vi "eyecat MAX v01_Js.vi"() -> ()   [LabVIEW 2011]
doc: "This VI is an upgrade from the WIN 1_v4 that implements the ageing subrutine"
uses:
  Buttons/String output.ctl
  <vilib>/Utility/miscctls.llb/LVRowAndColumnTypeDef.ctl
  Buttons/Numeric control.ctl
  Buttons/String input.ctl
  Buttons/Numeric indicator.ctl
  Controls Win/Control 3.ctl
  <vilib>/Platform/TimedLoop/XDataNode/nitl_modes.ctl
  <vilib>/Platform/TimedLoop/XDataNode/timing_clust.ctl
  <vilib>/Platform/TimedLoop/XDataNode/wakeup.ctl
  <vilib>/Utility/file.llb/Write To Spreadsheet File (string).vi
  <vilib>/Utility/file.llb/Read From Spreadsheet File (string).vi
  <vilib>/Platform/TimedLoop/XDataNode/XDataNode.xnode
  <vilib>/regexp/Match Regular Expression.xnode
  <vilib>/Platform/TimedLoop/XDataNode/XDNodeRunTimeDep.lvlib
panel:
  out "Furnace temp 2":dbl
  out "output cluster":T2
  out "Full system?":bool
  out "Log interval (seconds)":T1
  in  "Flow rate Age":dbl
  in  "Inlet temp Age":dbl
  out "Stopped?":bool
  in  "Stop Cmd":T1
  out "Connected?":bool
  out "Error":dbl
  out "Iteration Duration":i64
  out "Finished Late? [i-1]":bool
  in  "stop TCP":bool
  in  "SO2 ppm":dbl
  out "Furnace temp 1":dbl
  out "stop 2":bool
  in  "Enum 1":i16=1
  in  "Acknowledge":bool
  out "Test number":u16
  out "Flag1":bool=TRUE
  out "EditPos Subc":T3
  out "Flag 2":bool=TRUE
  in  "Tab Control":T4(tab)
  out "Doors Unlocked":bool
  in  "Temperature Limit (°C)":T1=800.0 min=0.0 max=1200.0 step=1.0
  in  "Log Test Button":bool
  in  "File Name":T5
  in  "File Path":path=path "C:/DATA LOG"
  out "Fail":bool
  out "Pass":bool
  in  "Select Test Type":T6(radio)
  out "Standby":bool
  out "Doors Open":bool
  out "Extractor Fan On":bool
  out "Test In Progress":bool
  out "Cool Down":bool
  out "System Alarm":bool
  in  "Execute Leak Test Button":bool
  in  "Stop Test Button":bool
  in  "Start Test Button":bool
  in  "Advanced settings":bool
  in  "Inlet Temperature (°C)":T1=400.0 min=350.0 max=1000.0 step=1.0
  in  "Inlet LAMBDA Rich":T1=0.9 min=0.85 max=0.96 step=0.001
  in  "Inlet LAMBDA Lean":T1=1.2 min=1.02 max=3.0 step=0.001
  in  "Test Stop temperature (°C)":T1=300.0 min=100.0 max=1000.0 step=1.0
  in  "Test Start Temperature (°C)":T1=125.0 min=0.0 max=500.0 step=1.0
  in  "Furnace Ramp Rate (°C/min)":T1=15.0 min=1.0 max=50.0 step=0.1
  in  "NO:CO Ratio":T1=1.1 min=1.0 max=5.0 step=0.1
  in  "Inlet O2 (%)":T1=0.5 min=0.0 max=14.0 step=0.01
  in  "Inlet LAMBDA":T1=1.0 min=0.6 max=3.0 step=0.001
  out "Space Velocity (h-1)":T7
  out "Vol Flow @ STP (l/min)":T7
  in  "Test Flow Rate(g/s)":T1 min=0.0 max=100.0 step=0.01
  out "Sample Volume (litres)":T7
  in  "Number of Samples":T1=1.0 min=1.0 max=6.0 step=1.0
  in  "Sample Diameter (mm)":T1
  out "CO Theory (%)":T7 format="%#_3g"
  out "CO Theory (%)":T7 format="%#_3g"
  out "HC Theory (%)":T7
  in  "Sample Length (mm)":T1 min=0.0 step=0.5
  in  "NO ppm SW":dbl=500.0 caption="NO (ppm)" min=0.0 max=500.0 step=1.0
  in  "NO ppm Loff":T1 caption="NO ppm"
  in  "Delete sCycle":bool
  in  "Load sCycle":bool
  in  "Save sCycle":bool
  in  "Clear subcycle":bool
  in  "Clear Cycle Pattern":bool
  in  "Save Cycle":bool
  in  "Load Cycle":bool
  in  "Delete Cycle":bool
  out "Test Compiled":bool
  in  "Compile Test Button":bool
  in  "Sub-Cycle List":i32(listbox)=1
  in  "Cycle List":i32(listbox)=2
  out "Total Test Duration (hrs)":T8
  in  "Ageing Gas":enum32{"Radio Selection 1", "Radio Selection 2"}(radio)
  in  "Sub-Cycle Pattern":string[][](table) caption="Subcycle pattern"
  in  "Total Number of Cycles":T1=1.0 min=1.0 max=10000.0 step=1.0
  in  "Cycle Pattern":string[][](table)
  in  "Sub-Cycle Name":T5
  in  "Cycle Name":T5
  out "Heat Exchanger Temperatures (°C)":dynamicdata(graph)
  out "Flow Rate (g/s)":dynamicdata(graph)
  out "Sample Temperatures (°C)":dynamicdata(graph)
  out "System Temperatures (°C)":dynamicdata(graph)
  out "HC Concentration (ppm)":dynamicdata(graph)
  out "Lambda":dynamicdata(graph)
  out "M584L Upstream & Downstream":dynamicdata(graph)
  out "NO Concentration (ppm)":dynamicdata(graph)
  in  "Purge System":bool
  in  "Alarm ack":bool
  in  "Clear log":bool
  out "Table":string[][](table)
  out "Soft Alarm":bool
  out "Hard Alarm":bool
  # "Test Type"
  # "Test Commands"
  # "System Indicators"
  # "Leak Test"
  # "Catalyst Specification"
  # "Lightoff Settings"
  # "Furnace Lightoff Settings"
  # "Sweep Settings"
  # "CO/HC Lightoff Settings"
  # "0.96 < lambda < 0.85"
  # "1.02< lambda < 1.6"
  # "350 < Tinlet < 1000"
  # "NO Lightoff Settings"
  # "Flow Specification"
  # "Cycle Compiled"
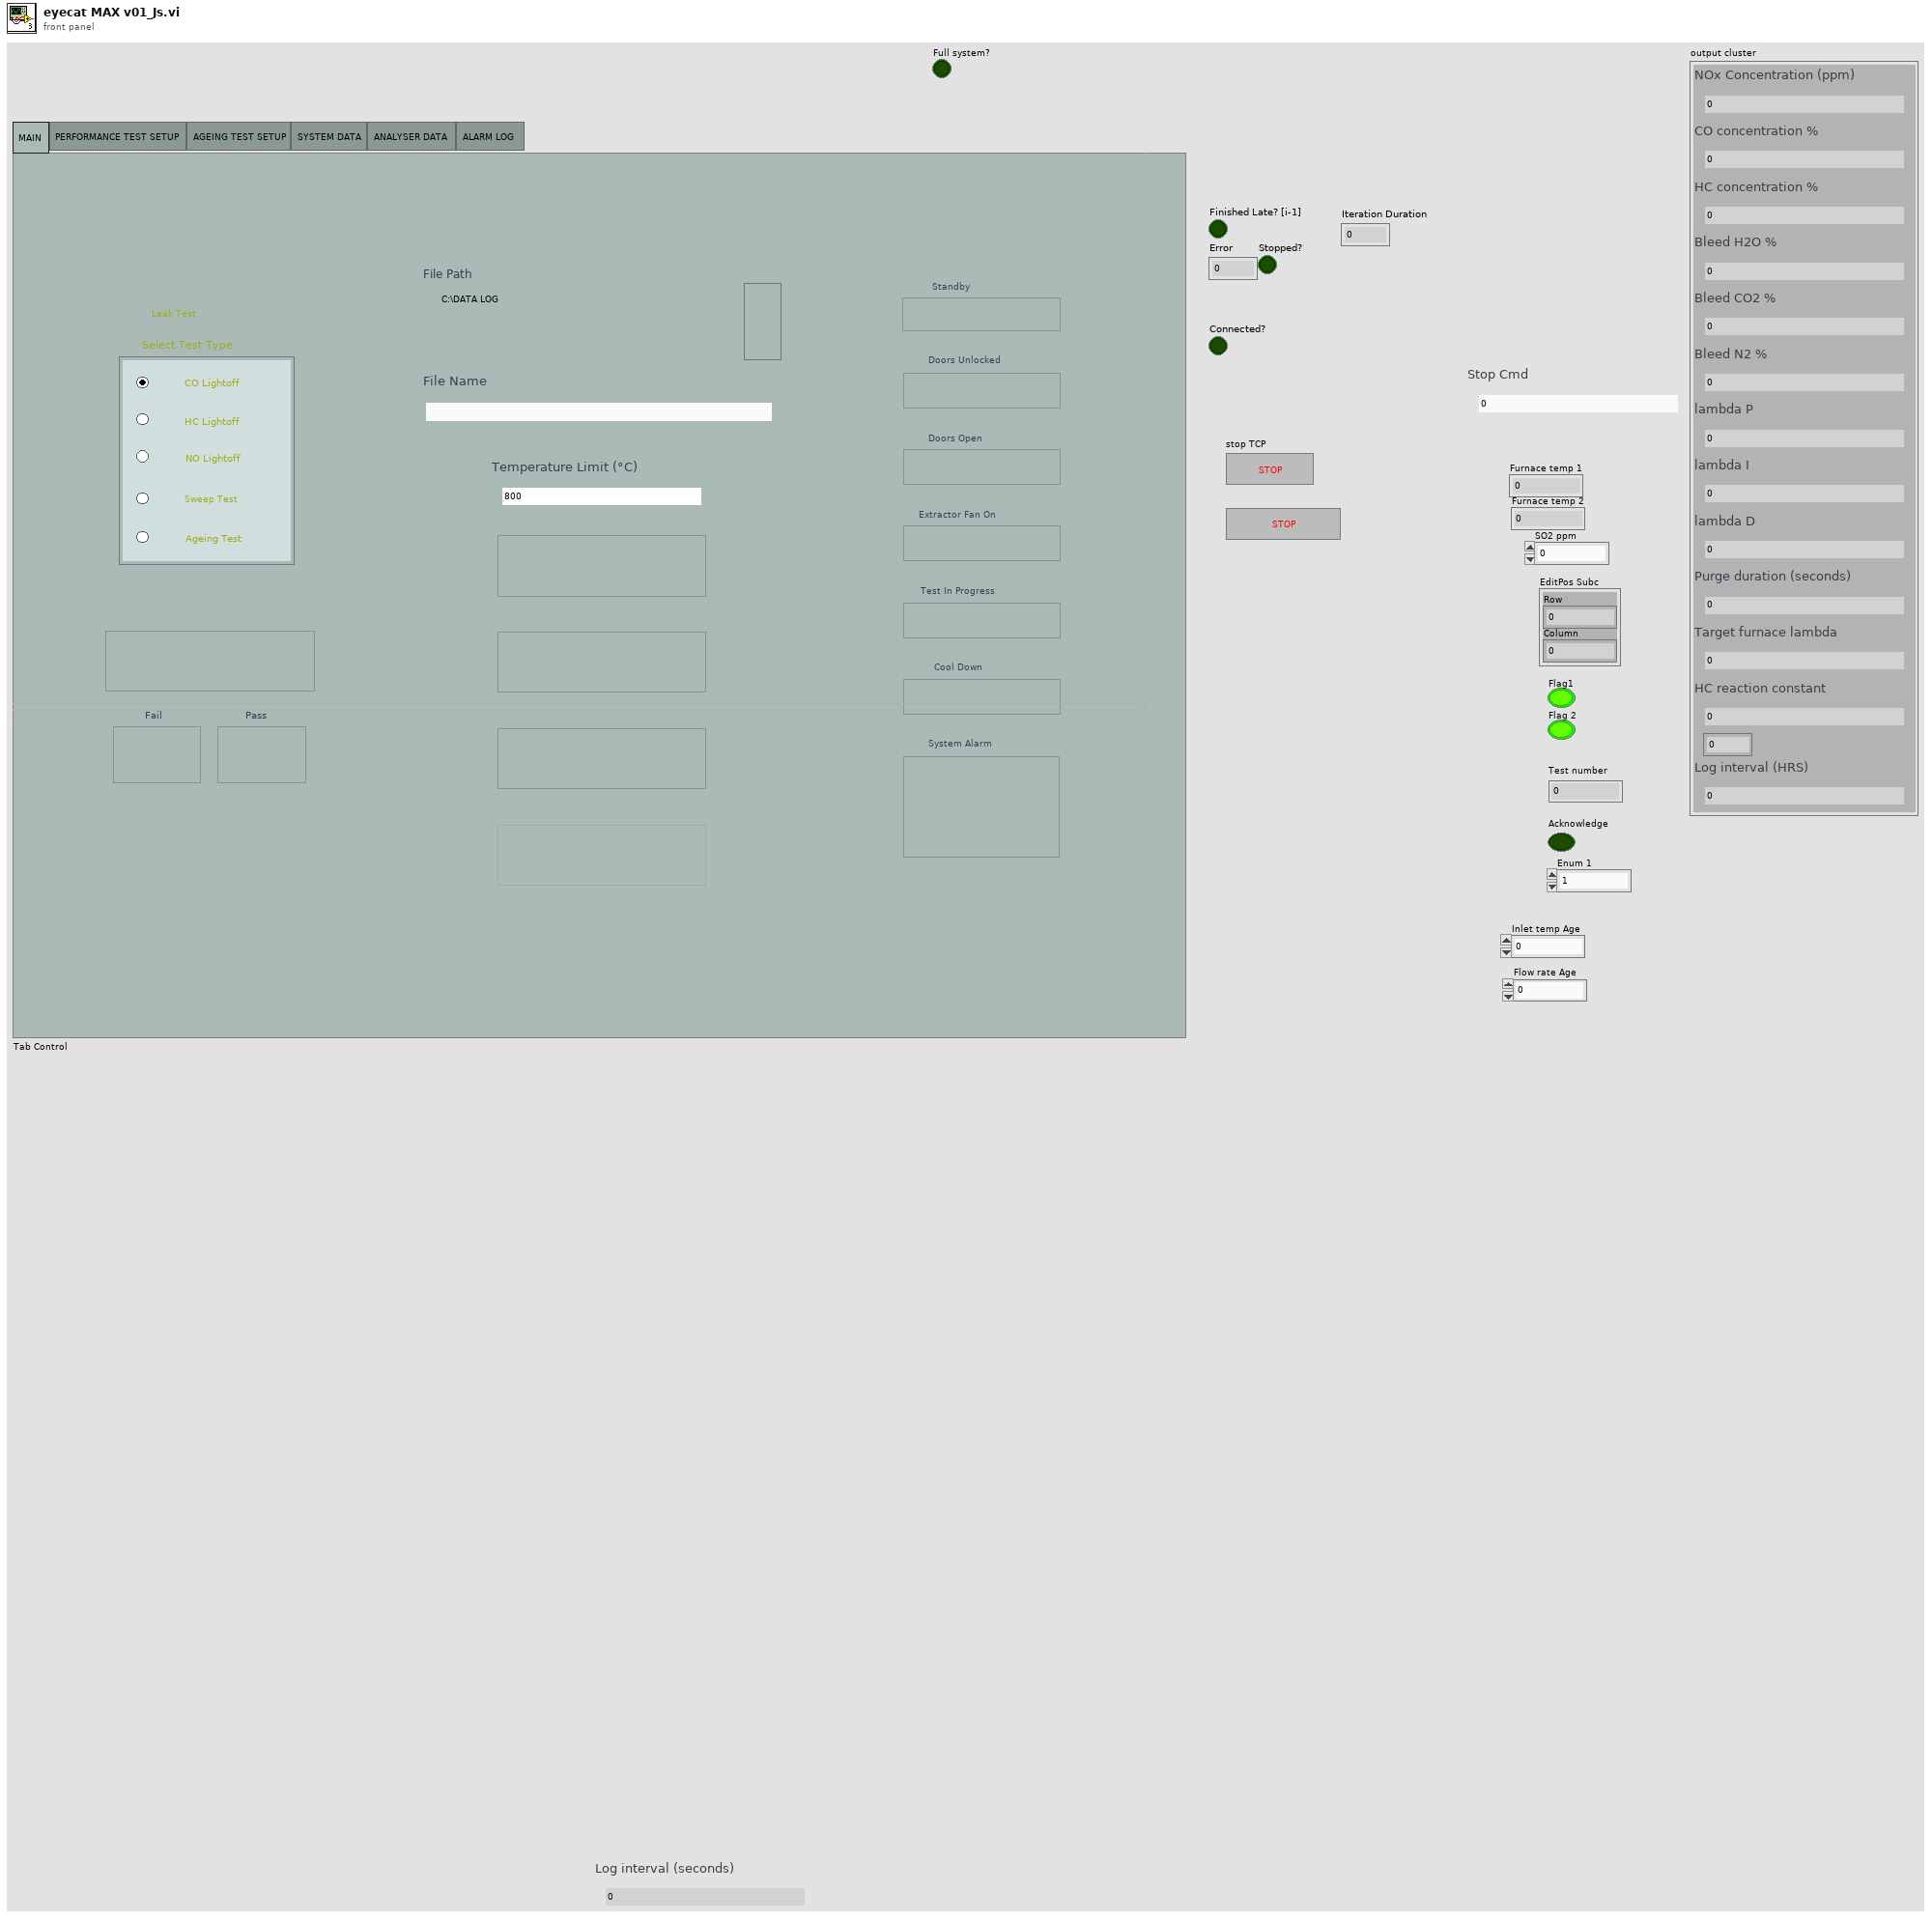
[diagram p1: front panel]
types:
  T1 = typedef "Numeric control.ctl" = dbl
  T2 = cluster{"NOx Concentration (ppm)":T1, "CO concentration %":T1, "HC concentration %":T1, "Bleed H2O %":T1, "Bleed CO2 %":T1, "Bleed N2 %":T1, "lambda P":T1, "lambda I":T1, "lambda D":T1, "Purge duration (seconds)":T1, "Target furnace lambda":T1, "HC reaction constant":T1, i16, "Log interval (HRS)":T1}
  T3 = typedef "LVRowAndColumnTypeDef.ctl" = cluster{"Row":i32, "Column":i32}
  T4 = enum32{"MAIN", "PERFORMANCE TEST SETUP", "AGEING TEST SETUP", "SYSTEM DATA", "ANALYSER DATA", "ALARM LOG"}
  T5 = typedef "String input.ctl" = string
  T6 = enum32{"CO Lightoff", "HC Lightoff", "NO Lightoff", "Sweep Test", "Ageing Test"}
  T7 = typedef "Numeric indicator.ctl" = dbl
  T8 = typedef "String output.ctl" = string
  T9 = typedef "XDNodeRunTimeDep.lvlib/nitl_modes.ctl" = enum32{"No Change", "Process missed periods, maintain original phase", "Discard missed periods, maintain original phase", "Process missed periods, ignore original phase", "Discard missed periods, ignore original phase"}
  T10 = typedef "Control 3.ctl" = enum16{"main", "start test", "save subc", "load subc", "delete subc", "clear table 1", "update list 1", "save cycle", "load cycle", "delete cycle", "clear table 2", "update list 2", "calc HC CO", "Total time calc", "update Cycle pattern ", "load cycle name", "convert to num", "load test array", "check scycle name", "check cycle name", "Multigas connect", "Multigas disconnect"}
  T11 = typedef "XDNodeRunTimeDep.lvlib/timing_clust.ctl" = cluster{"Expected End [f-1]":u64, "Actual End [f-1]":u64, "Finished Late? [f-1]":bool, "Expected End [i-1]":u64, "Actual End [i-1]":u64, "Finished Late? [i-1]":bool, "Expected Start [i]":u64, "Actual Start [i]":u64, "Expected Start [f]":u64, "Actual Start [f]":u64, "Source Name":string, "Structure Name":string, "Period":i64, "Deadline":i64, "Offset":i64, "Start":i64, "Priority":i32, "Timeout":i32, "Mode":T9, "Wakeup Reason":T12, "Error":errorcluster, "Source Type":string, "Secondary Source Type":string, "Global End Time":u64, "Global Start Time":u64, "Frame Duration":u64, "Iteration Duration":u64, "Assigned CPU":i32, "I/O Scan Engine Mode":u32}
  T12 = typedef "XDNodeRunTimeDep.lvlib/wakeup.ctl" = enum32{"Normal", "Aborted", "Asynchronous wakeup", "Timing source error", "Timed loop error", "Timeout"}
  T13 = enum8{"Enabled", "Disabled", "Disabled and Grayed Out"}
  T14 = cluster{"NOx Concentration (ppm)":T1, "CO concentration %":T1, "HC concentration %":T1, "Bleed H2O %":T1, "Bleed CO2 %":T1, "Bleed N2 %":T1, "lambda P":T1, "lambda I":T1, "lambda D":T1, "Purge duration (seconds)":T1, "Target furnace lambda":T1, "HC reaction constant":T1, "Full System?":i16, "Log interval (HRS)":T1}
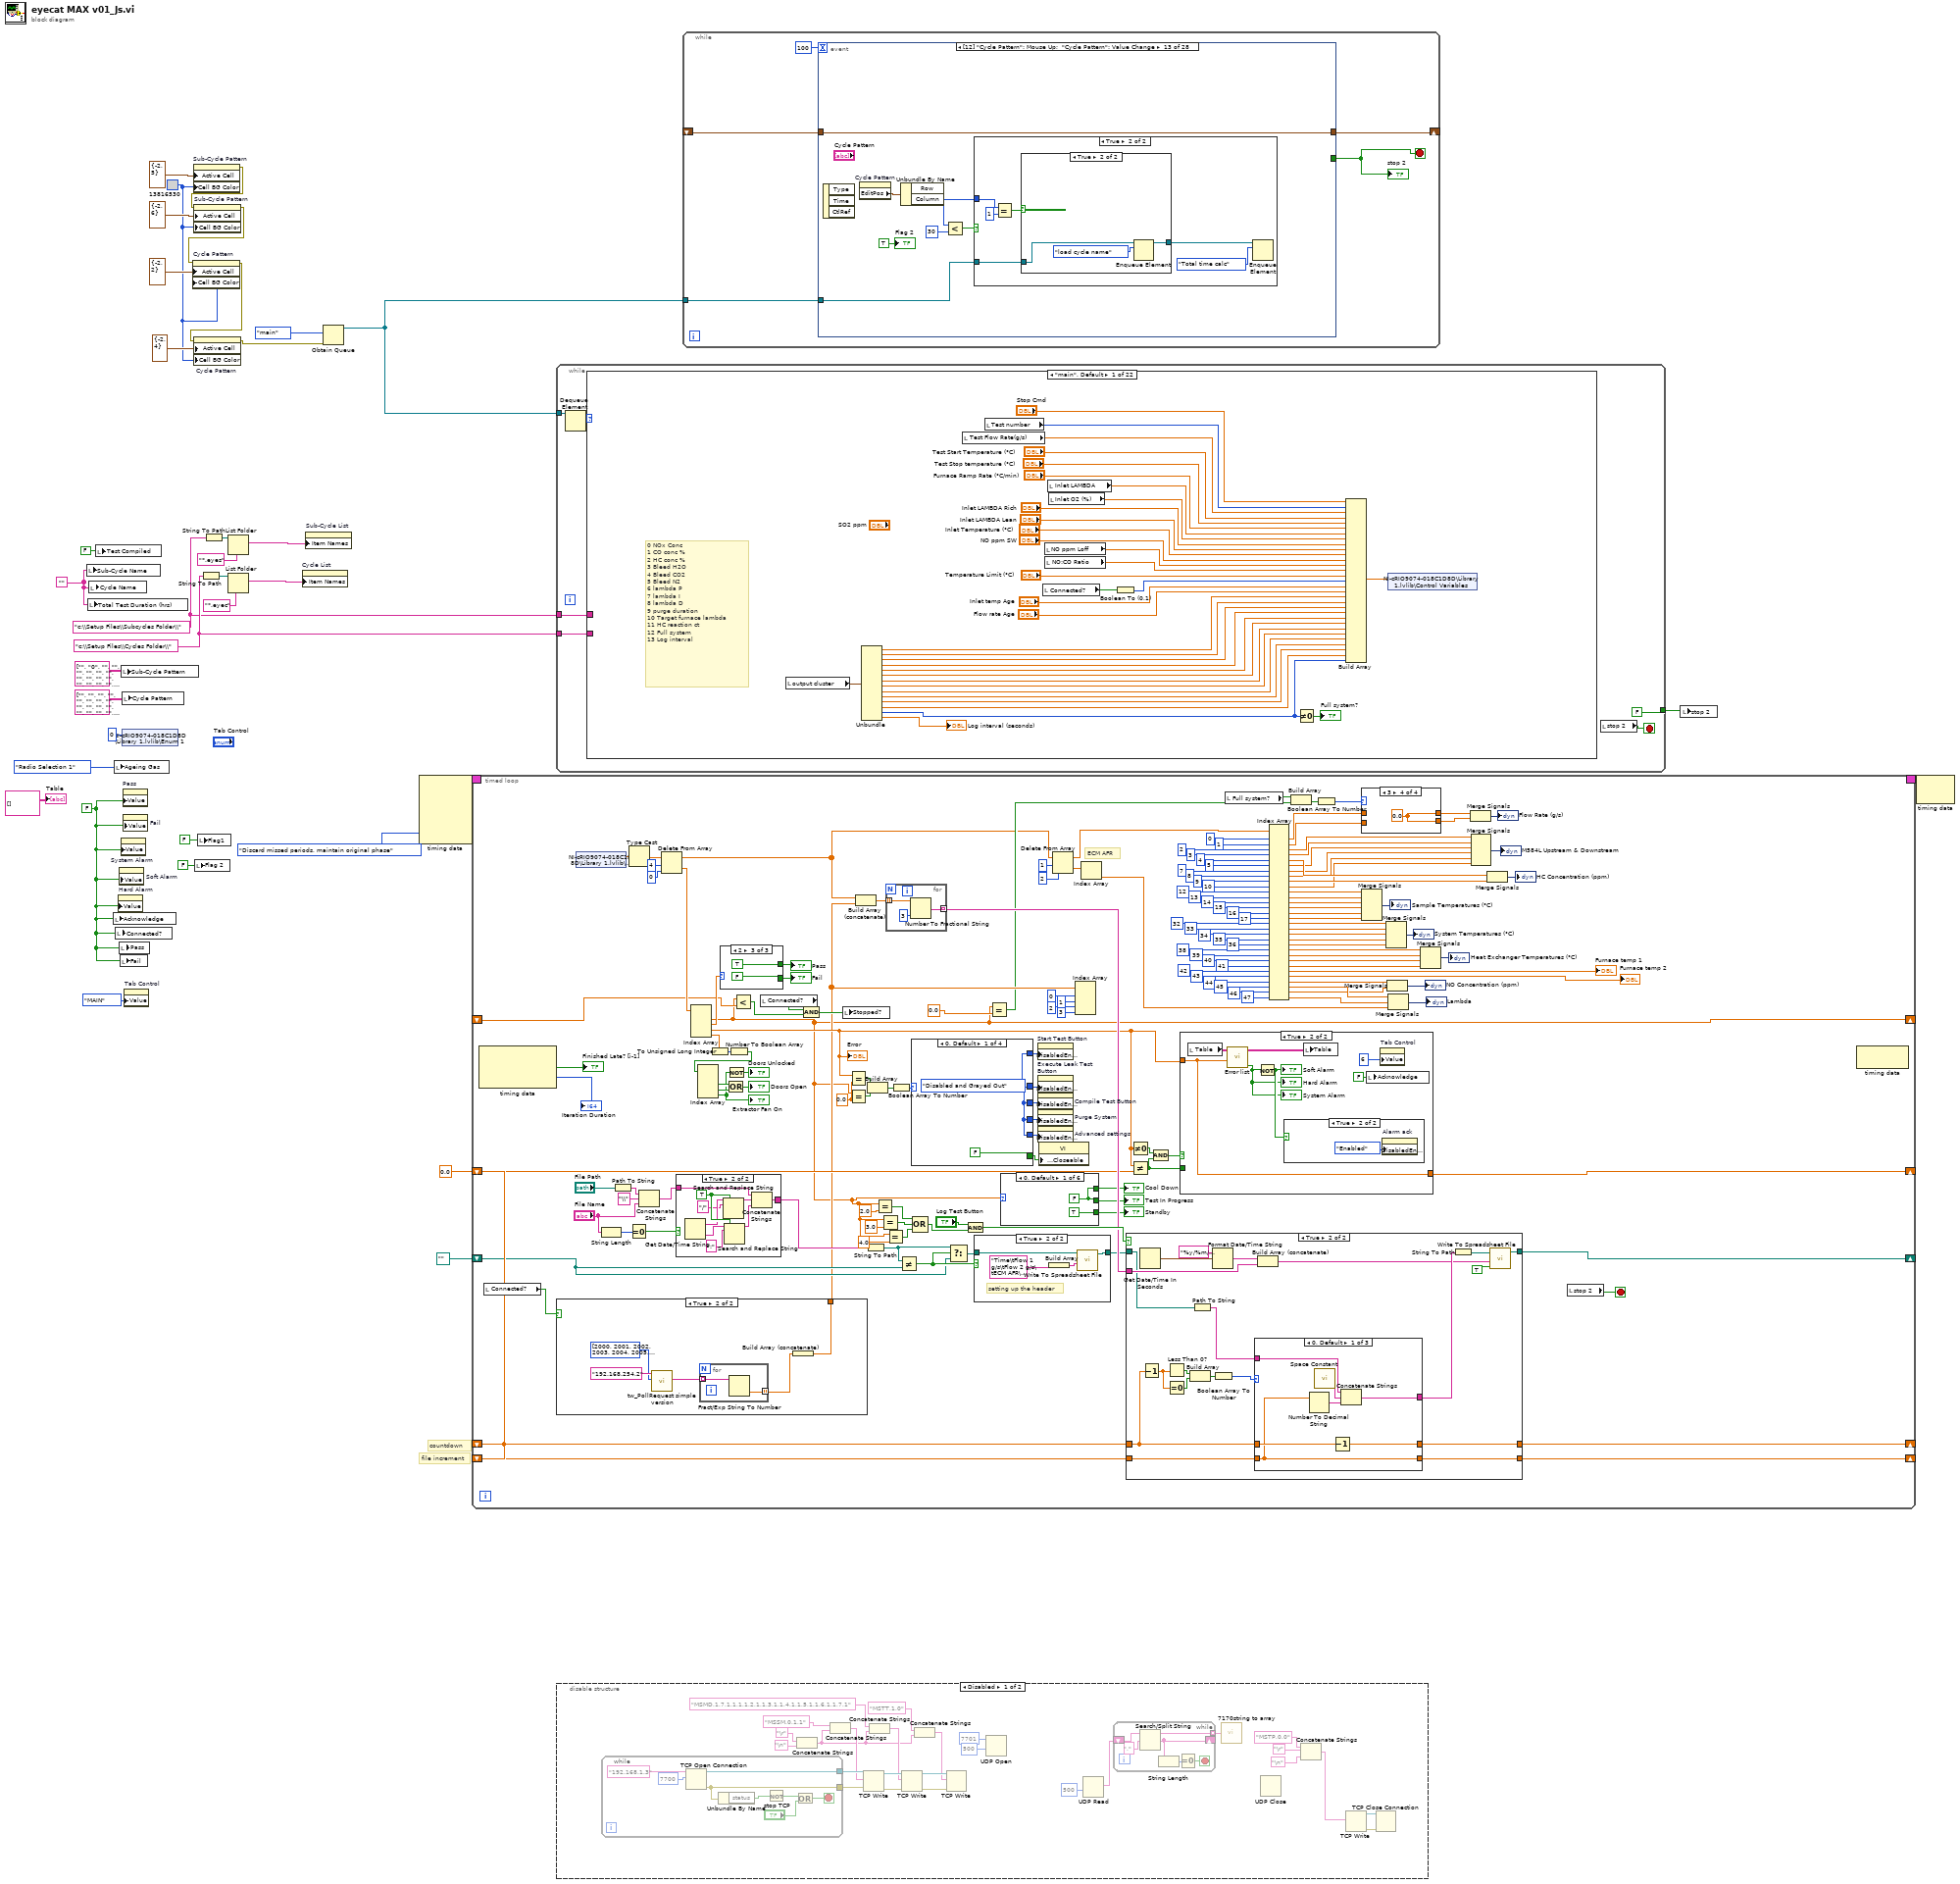
[diagram p0: block diagram]
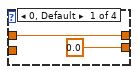
[diagram p3: hidden frame]
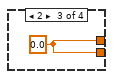
[diagram p5: hidden frame]
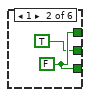
[diagram p7: hidden frame]
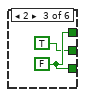
[diagram p8: hidden frame]
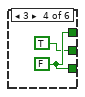
[diagram p9: hidden frame]
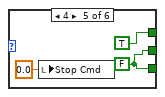
[diagram p10: hidden frame]
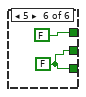
[diagram p11: hidden frame]
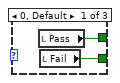
[diagram p12: hidden frame]
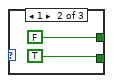
[diagram p13: hidden frame]
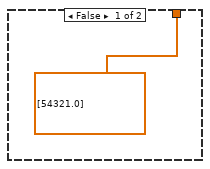
[diagram p14: hidden frame]
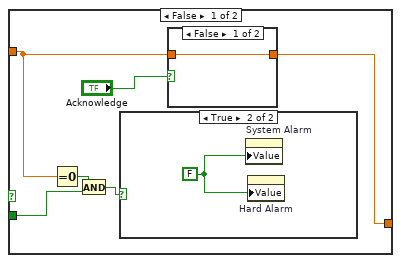
[diagram p15: hidden frame]
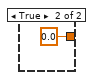
[diagram p16: hidden frame]
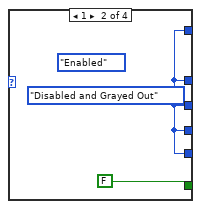
[diagram p19: hidden frame]
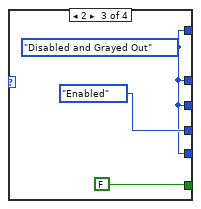
[diagram p20: hidden frame]
diagram:
  w2 = FALSE
  w1 = 0.0 ("y")
  w18 = ""
  w21 = "c:\\Setup Files\\Cycles Folder\\"
  w27 = u32 13816530
  w19 = "c:\\Setup Files\\Subcycles Folder\\"
  # "file increment"
  # "countdown"
  n1 = local write "Sub-Cycle Name"(w18) -> ()
  n2 = local write "Total Test Duration (hrs)"(w18) -> ()
  n3 = local write "Cycle Name"(w18) -> ()
  n4 = local write "Test Compiled"(FALSE ("Cycle Compiled")) -> ()
  n5 = local write "Acknowledge"(w2) -> ()
  n6 = local write "Ageing Gas"(enum32{"Radio Selection 1", "Radio Selection 2"}."Radio Selection 1" ("Ageing Gas")) -> ()
  n7 = local write "Connected?"(w2) -> ()
  n8 = property on="Hard Alarm" class="Bool (strict)"("Value"=w2) -> ()  [unwired: 2 in, 2 out]
  n9 = property on="Soft Alarm" class="Bool (strict)"("Value"=w2) -> ()  [unwired: 2 in, 2 out]
  n10 = local write "Pass"(w2) -> ()
  n11 = local write "Fail"(w2) -> ()
  n12 = local write "Sub-Cycle Pattern"(string[][] [["", "0", "", "", "", "", "", "", "", "", "", "", ""], ["", "", "", "", "", "", "", "", "", "", "", "", ""], ["", "", "", "", "", "", "", "", "", "", "", "", ""], ["", "", "", "", "", "", "", "", "", "", "", "", ""], ["", "", "", "", "", "", "", "", "", "", "", "", ""], ["", "", "", "", "", "", "", "", "", "", "", "", ""], ["", "", "", "", "", "", "", "", "", "", "", "", ""], ["", "", "", "", "", "", "", "", "", "", "", "", ""], ["", "", "", "", "", "", "", "", "", "", "", "", ""], ["", "", "", "", "", "", "", "", "", "", "", "", ""], ["", "", "", "", "", "", "", "", "", "", "", "", ""], ["", "", "", "", "", "", "", "", "", "", "", "", ""], ["", "", "", "", "", "", "", "", "", "", "", "", ""], ["", "", "", "", "", "", "", "", "", "", "", "", ""], ["", "", "", "", "", "", "", "", "", "", "", "", ""], ["", "", "", "", "", "", "", "", "", "", "", "", ""], ["", "", "", "", "", "", "", "", "", "", "", "", ""], ["", "", "", "", "", "", "", "", "", "", "", "", ""], ["", "", "", "", "", "", "", "", "", "", "", "", ""], ["", "", "", "", "", "", "", "", "", "", "", "", ""], ["", "", "", "", "", "", "", "", "", "", "", "", ""], ["", "", "", "", "", "", "", "", "", "", "", "", ""], ["", "", "", "", "", "", "", "", "", "", "", "", ""], ["", "", "", "", "", "", "", "", "", "", "", "", ""], ["", "", "", "", "", "", "", "", "", "", "", "", ""], ["", "", "", "", "", "", "", "", "", "", "", "", ""], ["", "", "", "", "", "", "", "", "", "", "", "", ""], ["", "", "", "", "", "", "", "", "", "", "", "", ""], ["", "", "", "", "", "", "", "", "", "", "", "", ""], ["", "", "", "", "", "", "", "", "", "", "", "", ""], ["", "", "", "", "", "", "", "", "", "", "", "", ""]]) -> ()
  n13 = property on="System Alarm" class="Bool (strict)"("Value"=w2) -> ()  [unwired: 2 in, 2 out]
  n14 = local write "Cycle Pattern"(string[][] [["", "", "", "", ""], ["", "", "", "", ""], ["", "", "", "", ""], ["", "", "", "", ""], ["", "", "", "", ""], ["", "", "", "", ""], ["", "", "", "", ""], ["", "", "", "", ""], ["", "", "", "", ""], ["", "", "", "", ""], ["", "", "", "", ""], ["", "", "", "", ""], ["", "", "", "", ""], ["", "", "", "", ""], ["", "", "", "", ""], ["", "", "", "", ""], ["", "", "", "", ""], ["", "", "", "", ""], ["", "", "", "", ""], ["", "", "", "", ""], ["", "", "", "", ""], ["", "", "", "", ""], ["", "", "", "", ""], ["", "", "", "", ""], ["", "", "", "", ""], ["", "", "", "", ""], ["", "", "", "", ""], ["", "", "", "", ""], ["", "", "", "", ""], ["", "", "", "", ""], ["", "", "", "", ""]]) -> ()
  n15 = shared-variable "NI-cRIO9074-018C1D8D\\Library 1.lvlib\\Enum 1"(u16 0 ("Enum 1")) -> ()  [unwired: 1 in, 1 out]
  n16 = property on="Pass" class="Bool (strict)"("Value"=w2) -> ()  [unwired: 2 in, 2 out]
  n17 = property on="Fail" class="Bool (strict)"("Value"=w2) -> ()  [unwired: 2 in, 2 out]
  n18 = property on="Tab Control" class="TabCtl (strict)"("Value"=T4."MAIN" ("Tab Control")) -> ()  [unwired: 2 in, 2 out]
  n19 = property on="Sub-Cycle Pattern" class="Tbl (strict)"("Active Cell"=T3 {"Row"=-2, "Column"=5} ("Active Cell:Active Cell"), "Cell BG Color"=w27) -> (error out=w32:errorcluster)  [unwired: 2 in, 1 out]
  n20 = property on="Sub-Cycle Pattern" class="Tbl (strict)"(error in=w32, "Active Cell"=T3 {"Row"=-2, "Column"=6} ("Active Cell:Active Cell"), "Cell BG Color"=w27) -> (error out=w31:errorcluster)  [unwired: 1 in, 1 out]
  n21 = property on="Cycle Pattern" class="Tbl (strict)"(error in=w31, "Active Cell"=T3 {"Row"=-2, "Column"=2} ("Active Cell:Active Cell"), "Cell BG Color"=w27) -> (error out=w29:errorcluster)  [unwired: 1 in, 1 out]
  n22 = property on="Cycle Pattern" class="Tbl (strict)"(error in=w29, "Active Cell"=T3 {"Row"=-2, "Column"=4} ("Active Cell:Active Cell"), "Cell BG Color"=w27) -> (error out=w26:errorcluster)  [unwired: 1 in, 1 out]
  n23 = local write "Flag 2"(FALSE) -> ()
  n24 = local write "Flag1"(FALSE) -> ()
  n25 = String To Path(string=w21) -> (path=w22:path)
  n26 = String To Path(string=w19) -> (path=w24:path)
  n27 = List Folder(path=w22, pattern="*.eyec") -> (filenames=w23:string[])  [unwired: 2 in, 3 out]
  n28 = List Folder(path=w24, pattern="*.eyes") -> (filenames=w25:string[])  [unwired: 2 in, 3 out]
  n29 = property on="Cycle List" class="LstBox (strict)"("Item Names"=w23) -> ()  [unwired: 2 in, 2 out]
  n30 = property on="Sub-Cycle List" class="LstBox (strict)"("Item Names"=w25) -> ()  [unwired: 2 in, 2 out]
  n31 = Obtain Queue(element data type=Control_3."main" ("Enum"), error in (no error)=w26) -> (queue out=w35:refnum<queue>)  [unwired: 3 in, 2 out]
  n32 = node-c288(nitl_modes."Discard missed periods, maintain original phase" ("Mode")) -> (w7:T11)  [unwired: 4 in]
  n33 = timed-loop {
    timing: w7 -> [_]
    timing-out: [_] -> w6
    shift-right: [w168] -> _
    shift-left: path "" -> [w170]
    shift-right: [w119] -> _
    shift-left: w1 -> [w169]
    shift-right: [w38] -> _
    shift-left: _ -> [w133]
    shift-right: [w108] -> _
    shift-left: w1 -> [w112]
    shift-right: [w109] -> _
    shift-left: w1 -> [w111]
    stop <- w167 stop-if-true
    w150 = 0.0 ("y")
    # "ECM AFR"
    n34 = node-c288() -> (→"Finished Late? [i-1]":bool, →"Iteration Duration":i64)  [unwired: 1 in, 1 out]
    n35 = local read "Connected?"() -> (w156:bool)
    n36 = case shown="True" w156 {
      tunnel: [dbl[] [54321.0] ("Output") w235] -> w107
      frame False {
      }
      frame True {
        n37 = call <userlib>:"tw_PollRequest simple version.vi"("EVID list"=i32[] [2000, 2001, 2002, 2003, 2004, 2005, 2006, 2007, 2008, 2009, 2010, 2011, 2012, 2013, 2014], "IP_ADD [127.0.0.1]"="192.168.254.2") -> ("values out"=w239:string[])  [unwired: 7 in, 2 out]
        n38 = for {
          tunnel: [w241] -> w236 mode=indexing
          tunnel: w239 -> [w240] mode=indexing
          n39 = Fract/Exp String To Number(string=w240) -> (number=w241:dbl)  [unwired: 3 in, 1 out]
        }
        n40 = Build Array (concatenate)(w236) -> (w235:dbl[])
      }
    }
    n41 = shared-variable "NI-cRIO9074-018C1D8D\\Library 1.lvlib\\DATA"() -> (w166:dbl[])  [unwired: 1 in, 1 out]
    n42 = String Length(string="File Name") -> (length=w124:i32)
    n43 = Path To String(path="File Path") -> (string=w126:string)
    n44 = Equal To 0?(x=w124) -> (x = 0?=w122:bool)
    n45 = Type Cast(type=w166, x=w166) -> (*(type *) &x=w179:dbl[])
    n46 = Concatenate Strings(w126, "\\" ("string"), "File Name") -> (w121:string)
    n47 = Delete From Array(array=w179, length=4, index=0) -> (deleted portion=w176:dbl[], array with subset deleted=w48:dbl[])
    n48 = case shown="True" w122 {
      tunnel: [w205 w213] -> w110
      tunnel: w121 -> [w205 w214]
      frame False {
      }
      frame True {
        w211 = TRUE ("replace all? (F)")
        n49 = Get Date/Time String() -> (date string=w209:string, time string=w210:string)  [unwired: 3 in]
        n50 = Search and Replace String(replace all?=w211, input string=w209, search string="/") -> (result string=w212:string)  [unwired: 5 in, 3 out]
        n51 = Search and Replace String(replace all?=w211, input string=w210, search string=":") -> (result string=w206:string)  [unwired: 5 in, 3 out]
        n52 = Concatenate Strings(w214, w212, w206) -> (w213:string)
      }
    }
    n53 = Index Array(array=w176) -> (element #1=w38:dbl, element #2=w139:dbl, element #3=w140:dbl, element #4=w132:dbl)  [unwired: 4 in]
    "Error" <- w140
    n54 = To Unsigned Long Integer(number=w132) -> (unsigned 32bit integer=w131:u32)
    n55 = case shown="2" w139 {
      tunnel: [w228 TRUE FALSE] -> w138
      tunnel: [w229 FALSE TRUE] -> w137
      frame 0, Default {
        n56 = local read "Pass"() -> (w229:bool)
        n57 = local read "Fail"() -> (w228:bool)
      }
      frame 1 {
      }
      frame 2 {
      }
    }
    "Pass" <- w137
    "Fail" <- w138
    n58 = Number To Boolean Array(number=w131) -> (Boolean array=w155:bool[])
    n59 = Index Array(array=w155) -> (element #2=w153:bool, element #3=w152:bool, element #4=w128:bool)  [unwired: 4 in, 1 out]
    "Extractor Fan On" <- w128
    n60 = Or(x=w153, y=w152) -> (x .or. y?=→"Doors Open":bool)
    n61 = Not(x=w128) -> (.not. x?=→"Doors Unlocked":bool)
    n62 = Less?(x=w38, y=w133) -> (x < y?=w130:bool)
    n63 = local read "Connected?"() -> (w129:bool)
    n64 = And(x=w129, y=w130) -> (x .and. y?=w118:bool)
    n65 = local write "Stopped?"(w118) -> ()
    n66 = Equal?(x=w140, y=w150) -> (x = y?=w148:bool)
    n67 = Equal?(x=w38, y=w150) -> (x = y?=w147:bool)
    n68 = Build Array (concatenate)(w48, w107) -> (w172:dbl[])
    n69 = String To Path(string=w110) -> (path=w120:path)
    n70 = Build Array(w148, w147) -> (w146:bool[])
    n71 = Equal?(x=w38, y=2.0) -> (x = y?=w50:bool)
    n72 = Equal?(x=w38, y=3.0) -> (x = y?=w41:bool)
    n73 = Equal?(x=w38, y=4.0) -> (x = y?=w39:bool)
    n74 = for {
      tunnel: w172 -> [w274] mode=indexing
      tunnel: [w273] -> w183 mode=indexing
      n75 = Number To Fractional String(number=w274, precision (6)=i16 3) -> (F-format string=w273:string)  [unwired: 2 in]
    }
    n76 = Boolean Array To Number(Boolean array=w146) -> (number=w145:u32)
    n77 = Not Equal?(x=w120, y=w170) -> (x != y?=w181:bool)
    n78 = case shown="0, Default" w145 {
      tunnel: [w260 w262 w264 w267] -> w149
      tunnel: [w260 w262 w264 w267] -> w144
      tunnel: [w260 w262 w264 w267] -> w143
      tunnel: [w260 w262 T13."Enabled" ("Disabled") w267] -> w142
      tunnel: [w260 w262 w264 w267] -> w141
      tunnel: [FALSE FALSE FALSE TRUE] -> w117
      frame 0, Default {
        w260 = T13."Disabled and Grayed Out" ("Disabled")
      }
      frame 1 {
        (unwired) T13."Enabled" ("Disabled")
        w262 = T13."Disabled and Grayed Out" ("Disabled")
      }
      frame 2 {
        w264 = T13."Disabled and Grayed Out" ("Disabled")
      }
      frame 3 {
        w267 = T13."Enabled" ("Disabled")
        (unwired) T13."Disabled and Grayed Out" ("Disabled")
      }
    }
    n79 = Compound Arithmetic op=OR(w50, w41, w39) -> (w49:bool)
    n80 = Select(t=w120, s=w181, f=w170) -> (s? t:f=w182:path)
    n81 = And(x="Log Test Button", y=w49) -> (x .and. y?=w198:bool)
    n82 = case shown="True" w181 {
      tunnel: w182 -> [w268 w272]
      tunnel: [w268 w271] -> w180
      frame False {
      }
      frame True {
        # "setting up the header"
        n83 = Build Array("Time\tFlow 1 g/s\tFlow 2 g/s\tECM AFR\tCO2 U %\tCO U %\tHC U ppm\tO2 U %\tNO U ppm\tCO2 D %\tCO D %\tHC D ppm\tO2 D %\tNO D ppm\tTC1X\tTC2A\tTCY\tTC4B\tTC5\tTC6\tTC7\tTC8\tTC9\tTC10\tTC11\tTC12\tTC13\tTC14\tTC15\tTC16\tTC17\tTC18\tTC19\tTC20\tTC Vent 1\tTC Vent 2\tTC Fan B1\tTC Fan B2\tTC Cab\tTC Ex A\tTC Ex B\tTC Ex C\tTC Ex D\tTC Furn 1\tTC Furn 2\tNOX 1 ppm\tNLambda 1\tNOX 2 ppm\tNLambda 2\tEGO 1\tEGO 2\tEGO 3\tEGO 4\tCO2 U %\tCO U %\tHC U ppm\tO2 U %\tNO U ppm\tCO2 D %\tCO D %\tHC D ppm\tO2 D %\tNO D ppm\r\n" ("Heading string 2")) -> (w270:string[])
        n84 = call-poly <vilib>:"Write To Spreadsheet File.vi"("1D data"=w270, "file path (dialog if empty)"=w272) -> ("new file path (Not A Path if cancelled)"=w271:path)  [unwired: 6 in]
      }
    }
    n85 = Equal?(x=w38, y=0.0) -> (x = y?=w104:bool)
    n86 = case shown="0, Default" w38 {
      tunnel: [w215 w218 w220 w222 TRUE FALSE] -> w136
      tunnel: [w215 TRUE TRUE TRUE w224 w226] -> w135
      tunnel: [TRUE w218 w220 w222 w224 w226] -> w134
      frame 0, Default {
        w215 = FALSE
      }
      frame 1 {
        w218 = FALSE
      }
      frame 2 {
        w220 = FALSE
      }
      frame 3 {
        w222 = FALSE
      }
      frame 4 {
        w224 = FALSE
        n87 = local write "Stop Cmd"(T1 0.0 ("Stop Cmd")) -> ()
      }
      frame 5 {
        w226 = FALSE
      }
    }
    "Cool Down" <- w136
    "Test In Progress" <- w135
    "Standby" <- w134
    n88 = property on="Start Test Button" class="Bool"("DisabledEnum"=w149) -> ()  [unwired: 2 in, 2 out]
    n89 = property on="Execute Leak Test Button" class="Bool"("DisabledEnum"=w144) -> ()  [unwired: 2 in, 2 out]
    n90 = property on="Compile Test Button" class="Bool"("DisabledEnum"=w143) -> ()  [unwired: 2 in, 2 out]
    n91 = property on="Purge System" class="Bool"("DisabledEnum"=w142) -> ()  [unwired: 2 in, 2 out]
    n92 = property on="Advanced settings" class="Bool"("DisabledEnum"=w141) -> ()  [unwired: 2 in, 2 out]
    n93 = property class="VI"("Front Panel.Closeable"=w117) -> ()  [unwired: 2 in, 2 out]
    n94 = Delete From Array(array=w48, length=1, index=2) -> (deleted portion=w45:dbl[], array with subset deleted=w43:dbl[])
    n95 = Index Array(array=w107, index #1=0 ("index"), index #2=1 ("index"), index #3=2 ("index"), index #4=3 ("index")) -> ()  [unwired: 4 out]
    n96 = Index Array(array=w45) -> (element=w44:dbl)  [unwired: 1 in]
    n97 = case shown="True" w198 {
      tunnel: w180 -> [w278 w286]
      tunnel: [w278 w298] -> w168
      tunnel: w183 -> [_ w294]
      tunnel: w112 -> [_ w287]
      tunnel: w111 -> [w277 w282]
      tunnel: [w277 w284] -> w109
      tunnel: [w276 w283] -> w108
      frame False {
        n98 = local read "Log interval (seconds)"() -> (w276:T1)
      }
      frame True {
        n99 = Get Date/Time In Seconds() -> (seconds since 1Jan1904=w295:timestamp)
        n100 = Decrement(x=w287) -> (x-1=w288:T1)
        n101 = Less Than 0?(x=w288) -> (x < 0?=w289:bool)
        n102 = Equal To 0?(x=w288) -> (x = 0?=w290:bool)
        n103 = Build Array(w289, w290) -> (w291:bool[])
        n104 = Path To String(path=w286) -> (string=w281:string)
        n105 = Format Date/Time String(time format string (%c)="%y/%m/%d %H:%M:%S", seconds (now)=w295) -> (date/time string=w296:string)  [unwired: 1 in]
        n106 = Boolean Array To Number(Boolean array=w291) -> (number=w292:u32)
        n107 = case shown="0, Default" w292 {
          tunnel: w287 -> [w305 w306 _]
          tunnel: [w304 w306 w309] -> w283
          tunnel: w281 -> [w303 w308 w312]
          tunnel: [w300 w308 w310] -> w285
          tunnel: [w299 w307 w311] -> w284
          tunnel: w282 -> [w299 w307 w315]
          frame 0, Default {
            n108 = Number To Decimal String(number=w299) -> (decimal integer string=w301:string)  [unwired: 1 in]
            n109 = call <vilib>:"Space Constant.vi"() -> ("String"=w302:string)
            n110 = Decrement(x=w305) -> (x-1=w304:T1)
            n111 = Concatenate Strings(w303, w302, w301) -> (w300:string)
          }
          frame 1 {
          }
          frame 2 {
            n112 = local read "Log interval (seconds)"() -> (w309:T1)
            n113 = Increment(x=w315) -> (x+1=w311:dbl)
            n114 = Number To Decimal String(number=w311) -> (decimal integer string=w313:string)  [unwired: 1 in]
            n115 = call <vilib>:"Space Constant.vi"() -> ("String"=w314:string)
            n116 = Concatenate Strings(w312, w314, w313) -> (w310:string)
          }
        }
        n117 = Build Array (concatenate)(w296, w294) -> (w280:string[])
        n118 = String To Path(string=w285) -> (path=w279:path)
        n119 = call-poly <vilib>:"Write To Spreadsheet File.vi"("append to file? (new file:F)"=TRUE, "1D data"=w280, "file path (dialog if empty)"=w279) -> ("new file path (Not A Path if cancelled)"=w298:path)  [unwired: 5 in]
      }
    }
    n120 = Not Equal To 0?(x=w140) -> (x != 0?=w174:bool)
    n121 = Not Equal?(x=w140, y=w169) -> (x != y?=w173:bool)
    n122 = And(x=w174, y=w173) -> (x .and. y?=w175:bool)
    n123 = case shown="True" w175 {
      tunnel: w140 -> [w243 w254]
      tunnel: w173 -> [w246 _]
      tunnel: [w242 w254] -> w119
      frame False {
        n124 = Equal To 0?(x=w243) -> (x = 0?=w247:bool)
        n125 = And(x=w247, y=w246) -> (x .and. y?=w245:bool)
        n126 = case shown="True" w245 {
          frame False {
          }
          frame True {
            w250 = FALSE ("Ack hard alarm!")
            n127 = property on="System Alarm" class="Bool (strict)"("Value"=w250) -> ()  [unwired: 2 in, 2 out]
            n128 = property on="Hard Alarm" class="Bool (strict)"("Value"=w250) -> ()  [unwired: 2 in, 2 out]
          }
        }
        n129 = case shown="False" "Acknowledge" {
          tunnel: [w248 0.0 ("Numeric")] -> w242
          tunnel: w243 -> [w248 _]
          frame False {
          }
          frame True {
          }
        }
      }
      frame True {
        n130 = local read "Table"() -> (w257:string[][])
        n131 = call "Error list.vi"("Error code"=w254, "Error array in"=w257) -> ("Hard alarm?"=w251:bool, "Error array out"=w256:string[][])  [unwired: 8 in]
        "Hard Alarm" <- w251
        "System Alarm" <- w251
        n132 = Not(x=w251) -> (.not. x?=w252:bool)
        "Soft Alarm" <- w252
        n133 = case shown="True" w252 {
          frame False {
          }
          frame True {
            n134 = property on="Alarm ack" class="Bool"("DisabledEnum"=T13."Enabled" ("Disabled")) -> ()  [unwired: 2 in, 2 out]
          }
        }
        n135 = local write "Table"(w256) -> ()
        n136 = local write "Acknowledge"(FALSE ("Acknowledge")) -> ()
        n137 = property on="Tab Control" class="TabCtl (strict)"("Value"=6) -> ()  [unwired: 2 in, 2 out]
      }
    }
    n138 = local read "Full system?"() -> (w105:bool)
    n139 = Index Array(array=w43, index #1=0 ("index"), index #2=1 ("index"), index #3=2 ("index"), index #4=3 ("index"), index #5=4 ("index"), index #6=5 ("index"), index #7=7 ("index"), index #8=8 ("index"), index #9=9 ("index"), index #10=10 ("index"), index #11=12 ("index"), index #12=13 ("index"), index #13=14 ("index"), index #14=15 ("index"), index #15=16 ("index"), index #16=17 ("index"), index #17=32 ("index"), index #18=33 ("index"), index #19=34 ("index"), index #20=35 ("index"), index #21=36 ("index"), index #22=38 ("index"), index #23=39 ("index"), index #24=40 ("index"), index #25=41 ("index"), index #26=42 ("index"), index #27=43 ("index"), index #28=44 ("index"), index #29=45 ("index"), index #30=46 ("index"), index #31=47 ("index")) -> (element #1=w102:dbl, element #2=w101:dbl, element #3=w98:dbl, element #4=w96:dbl, element #5=w97:dbl, element #6=w95:dbl, element #7=w94:dbl, element #8=w93:dbl, element #9=w92:dbl, element #10=w91:dbl, element #11=w86:dbl, element #12=w85:dbl, element #13=w84:dbl, element #14=w83:dbl, element #15=w82:dbl, element #16=w81:dbl, element #17=w75:dbl, element #18=w74:dbl, element #19=w73:dbl, element #20=w72:dbl, element #21=w71:dbl, element #22=w66:dbl, element #23=w65:dbl, element #24=w64:dbl, element #25=w63:dbl, element #26=→"Furnace temp 1":dbl, element #27=→"Furnace temp 2":dbl, element #28=w56:dbl, element #29=w55:dbl, element #30=w52:dbl, element #31=w51:dbl)
    n140 = Build Array(w105, w104) -> (w106:bool[])
    n141 = Boolean Array To Number(Boolean array=w106) -> (number=w103:u32)
    n142 = case shown="3" w103 {
      tunnel: w102 -> [w200 w202 _ _]
      tunnel: w101 -> [_ w201 _ _]
      tunnel: [w200 w202 w203 w204] -> w100
      tunnel: [0.0 ("y") w201 w203 w204] -> w99
      frame 0, Default {
      }
      frame 1 {
      }
      frame 2 {
        w203 = 0.0 ("y")
      }
      frame 3 {
        w204 = 0.0 ("y")
      }
    }
    n143 = Merge Signals(w86, w85, w84, w83, w82, w81) -> (→"Sample Temperatures (°C)":dynamicdata)
    n144 = Merge Signals(w75, w74, w73, w72, w71) -> (→"System Temperatures (°C)":dynamicdata)
    n145 = Merge Signals(w56, w52) -> (→"NO Concentration (ppm)":dynamicdata)
    n146 = Merge Signals(w55, w51, w44) -> (→"Lambda":dynamicdata)
    n147 = Merge Signals(w66, w65, w64, w63) -> (→"Heat Exchanger Temperatures (°C)":dynamicdata)
    n148 = Merge Signals(w100, w99) -> (→"Flow Rate (g/s)":dynamicdata)
    n149 = Merge Signals(w98, w96, w95, w94, w93, w91) -> (→"M584L Upstream & Downstream":dynamicdata)
    n150 = Merge Signals(w97, w92) -> (→"HC Concentration (ppm)":dynamicdata)
    n151 = local read "stop 2"() -> (w167:bool)
    n152 = node-c288() -> ()  [unwired: 1 in, 1 out]
  }
  n153 = while {
    tunnel: w35 -> [w324]
    tunnel: w19 -> [w322]
    tunnel: w21 -> [w321]
    tunnel: [FALSE ("stop 2")] -> w9
    stop <- w325 stop-if-true
    n154 = Dequeue Element(queue=w324) -> (element=w323:T10)  [unwired: 2 in, 3 out]
    n155 = case shown="\"main\", Default" w323 {
      tunnel: w322 -> [_ _ _ w370 w381 w417 w451 _ _ _ _ _ _ _ w814 _ _ _ _ _ _ _]
      tunnel: w321 -> [_ _ _ _ _ _ _ _ w464 w479 w534 w579 _ _ _ _ _ _ _ _ _ _]
      frame "main", Default {
        # "0 NOx Conc\n1 CO conc %\n2 HC conc %\n3 Bleed H2O \n4 Bleed CO2\n5 Bleed N2 \n6 lambda P\n7 lambda I\n8 lambda D\n9 purge duration\n10 Target furnace lambda\n11 HC reaction ct\n12 Full system\n13 Log interval"
        n156 = local read "output cluster"() -> (w344:T2)
        n157 = Unbundle(w344) -> ("NOx Concentration (ppm)"=w330:T1, "CO concentration %"=w329:T1, "HC concentration %"=w328:T1, "Bleed H2O %"=w327:T1, "Bleed CO2 %"=w326:T1, "Bleed N2 %"=w341:T1, "lambda P"=w340:T1, "lambda I"=w339:T1, "lambda D"=w342:T1, "Purge duration (seconds)"=w343:T1, "Target furnace lambda"=w335:T1, "HC reaction constant"=w334:T1, w336:i16, "Log interval (HRS)"=→"Log interval (seconds)":T1)
        n158 = local read "Test Flow Rate(g/s)"() -> (w356:T1)
        n159 = local read "Test number"() -> (w361:u16)
        n160 = local read "Connected?"() -> (w350:bool)
        n161 = local read "NO ppm Loff"() -> (w346:T1)
        n162 = local read "NO:CO Ratio"() -> (w345:T1)
        n163 = local read "Inlet LAMBDA"() -> (w348:T1)
        n164 = local read "Inlet O2 (%)"() -> (w347:T1)
        n165 = Boolean To (0,1)(Boolean=w350) -> (0, 1=w333:i16)
        n166 = Not Equal To 0?(x=w336) -> (x != 0?=→"Full system?":bool)
        n167 = Build Array("Stop Cmd", w361, w356, "Test Start Temperature (°C)", "Test Stop temperature (°C)", "Furnace Ramp Rate (°C/min)", w348, w347, "Inlet LAMBDA Rich", "Inlet LAMBDA Lean", "Inlet Temperature (°C)", "NO ppm SW", w346, w345, "Temperature Limit (°C)", w333, "Inlet temp Age", "Flow rate Age", w330, w329, w328, w327, w326, w341, w340, w339, w342, w343, w335, w334, w336) -> (w352:T1[])
        n168 = shared-variable "NI-cRIO9074-018C1D8D\\Library 1.lvlib\\Control Variables"(w352) -> ()  [unwired: 1 in, 1 out]
      }
      frame "start test" {
        w362 = FALSE
        n169 = property on="Pass" class="Bool (strict)"("Value"=w362) -> ()  [unwired: 2 in, 2 out]
        n170 = property on="Fail" class="Bool (strict)"("Value"=w362) -> ()  [unwired: 2 in, 2 out]
        n171 = local write "Pass"(w362) -> ()
        n172 = local write "Fail"(w362) -> ()
        n173 = shared-variable "NI-cRIO9074-018C1D8D\\Library 1.lvlib\\Enum 1"("Enum 1") -> ()  [unwired: 1 in, 1 out]
      }
      frame "clear table 1" {
        n174 = property on="Sub-Cycle Name" class="Str"("Value"="" ("Subcycle name")) -> ()  [unwired: 2 in, 2 out]
        n175 = local write "Flag1"(FALSE) -> ()
        n176 = local write "Sub-Cycle Pattern"(string[][] [["", "0", "", "", "", "", "", "", "", "", "", "", ""], ["", "", "", "", "", "", "", "", "", "", "", "", ""], ["", "", "", "", "", "", "", "", "", "", "", "", ""], ["", "", "", "", "", "", "", "", "", "", "", "", ""], ["", "", "", "", "", "", "", "", "", "", "", "", ""], ["", "", "", "", "", "", "", "", "", "", "", "", ""], ["", "", "", "", "", "", "", "", "", "", "", "", ""], ["", "", "", "", "", "", "", "", "", "", "", "", ""], ["", "", "", "", "", "", "", "", "", "", "", "", ""], ["", "", "", "", "", "", "", "", "", "", "", "", ""], ["", "", "", "", "", "", "", "", "", "", "", "", ""], ["", "", "", "", "", "", "", "", "", "", "", "", ""], ["", "", "", "", "", "", "", "", "", "", "", "", ""], ["", "", "", "", "", "", "", "", "", "", "", "", ""], ["", "", "", "", "", "", "", "", "", "", "", "", ""], ["", "", "", "", "", "", "", "", "", "", "", "", ""], ["", "", "", "", "", "", "", "", "", "", "", "", ""], ["", "", "", "", "", "", "", "", "", "", "", "", ""], ["", "", "", "", "", "", "", "", "", "", "", "", ""], ["", "", "", "", "", "", "", "", "", "", "", "", ""], ["", "", "", "", "", "", "", "", "", "", "", "", ""], ["", "", "", "", "", "", "", "", "", "", "", "", ""], ["", "", "", "", "", "", "", "", "", "", "", "", ""], ["", "", "", "", "", "", "", "", "", "", "", "", ""], ["", "", "", "", "", "", "", "", "", "", "", "", ""], ["", "", "", "", "", "", "", "", "", "", "", "", ""], ["", "", "", "", "", "", "", "", "", "", "", "", ""], ["", "", "", "", "", "", "", "", "", "", "", "", ""], ["", "", "", "", "", "", "", "", "", "", "", "", ""], ["", "", "", "", "", "", "", "", "", "", "", "", ""], ["", "", "", "", "", "", "", "", "", "", "", "", ""]]) -> ()
      }
      frame "update list 1" {
        n177 = String To Path(string=w370) -> (path=w369:path)
        n178 = List Folder(path=w369, pattern="*.eyes") -> (filenames=w368:string[])  [unwired: 2 in, 3 out]
        n179 = property on="Sub-Cycle List" class="LstBox (strict)"("Item Names"=w368) -> ()  [unwired: 2 in, 2 out]
      }
      frame "save subc" {
        w374 = ".eyes" ("string")
        n180 = local read "Sub-Cycle Name"() -> (w373:T5)
        n181 = String To Path(string=w381) -> (path=w386:path)
        n182 = Equal?(x=w373, y="") -> (x = y?=w378:bool)
        n183 = List Folder(path=w386, pattern="*.eyes" ("string")) -> (filenames=w385:string[])  [unwired: 2 in, 3 out]
        n184 = Concatenate Strings(w373, w374) -> (w372:string)
        n185 = Concatenate Strings(w381, w373, w374) -> (w387:string)
        n186 = Search 1D Array(1D array=w385, element=w372) -> (index of element=w384:i32)  [unwired: 1 in]
        n187 = case shown="True" w378 {
          tunnel: [TRUE FALSE] -> w377
          frame False {
          }
          frame True {
            n188 = One Button Dialog(message="Insert file name!") -> ()  [unwired: 1 in, 1 out]
          }
        }
        n189 = String To Path(string=w387) -> (path=w380:path)
        n190 = Equal?(x=w384, y=-1) -> (x = y?=w382:bool)
        n191 = case shown="False" w382 {
          selector: w382 -> [_ w393]
          tunnel: [w391 w393] -> w376
          frame False {
            n192 = Two Button Dialog(message="A file with this name already exists!\nDo you want to overwrite?") -> (T button?=w391:bool)  [unwired: 2 in]
          }
          frame True {
          }
        }
        n193 = And(x=w376, y=w377) -> (x .and. y?=w375:bool)
        n194 = case shown="True" w375 {
          tunnel: w380 -> [_ w398]
          frame False {
          }
          frame True {
            n195 = local read "Sub-Cycle Pattern"() -> (w397:string[][])
            n196 = call "Table check.vi"("Input table"=w397) -> ("Incomplete?"=w395:bool, "Length"=w396:i32)  [unwired: 9 in]
            n197 = case shown="False" w395 {
              tunnel: w397 -> [w406 _]
              tunnel: w398 -> [w405 _]
              tunnel: w396 -> [w404 _]
              tunnel: string[] [] -> [w403 _]
              frame False {
                n198 = for {
                  N: w404 -> [_]
                  tunnel: w406 -> [w413]
                  shift-right: [w410] -> w402
                  shift-left: w403 -> [w411]
                  i -> [w412]
                  n199 = Index Array(array=w413, index (row)=w412) -> (element=w409:string[])  [unwired: 1 in]
                  n200 = Delete From Array(array=w409, index=0) -> (array with subset deleted=w408:string[])  [unwired: 1 in, 1 out]
                  n201 = Build Array (concatenate)(w411, w408) -> (w410:string[])
                }
                n202 = Build Array (concatenate)("SubCycle Data File for EYECAT - do not modify", w402) -> (w400:string[])
                n203 = call-poly <vilib>:"Write To Spreadsheet File.vi"("1D data"=w400, "file path (dialog if empty)"=w405) -> ()  [unwired: 6 in, 1 out]
              }
              frame True {
                n204 = One Button Dialog(message="The table is incomplete!\nplease review and save again!") -> ()  [unwired: 1 in, 1 out]
              }
            }
            n205 = local write "Flag1"(FALSE) -> ()
          }
        }
      }
      frame "load subc" {
        n206 = local read "Flag1"() -> (w418:bool)
        n207 = case shown="True" w418 {
          tunnel: [w445 w447] -> w416
          tunnel: w417 -> [w445 w447]
          tunnel: [TRUE w446] -> w415
          frame False {
          }
          frame True {
            n208 = Two Button Dialog(message="The table has been modified.\nDo you want to continue?") -> (T button?=w446:bool)  [unwired: 2 in]
          }
        }
        n209 = case shown="True" w415 {
          tunnel: w416 -> [_ w422]
          frame False {
          }
          frame True {
            n210 = property on="Sub-Cycle List" class="LstBox (strict)"() -> ("Item Names"=w434:string[])  [unwired: 2 in, 2 out]
            n211 = Index Array(array=w434, index="Sub-Cycle List") -> (element=w421:string)
            n212 = Concatenate Strings(w422, w421) -> (w432:string)
            n213 = Search/Split String(string=w421, search string/char (-)=".") -> (substring before match=w419:string)  [unwired: 1 in, 2 out]
            n214 = local write "Sub-Cycle Name"(w419) -> ()
            n215 = String To Path(string=w432) -> (path=w431:path)
            n216 = call-poly <vilib>:"Read From Spreadsheet File.vi"("file path (dialog if empty)"=w431) -> ("first row"=w427:string[])  [unwired: 6 in, 4 out]
            n217 = Delete From Array(array=w427, length=1, index=0) -> (array with subset deleted=w424:string[])  [unwired: 1 out]
            n218 = Array Size(array=w424) -> (size(s)=w430:i32)
            n219 = Divide(x=w430, y=12) -> (x/y=w423:dbl)
            n220 = for {
              N: w423 -> [_]
              shift-right: [w440] -> _
              shift-left: w424 -> [w443]
              tunnel: [w439] -> w428 mode=indexing
              i -> [w438]
              n221 = Increment(x=w438) -> (x+1=w437:i32)
              n222 = Delete From Array(array=w443, length=12, index=0) -> (deleted portion=w435:string[], array with subset deleted=w440:string[])
              n223 = Number To Decimal String(number=w437) -> (decimal integer string=w436:string)  [unwired: 1 in]
              n224 = Build Array (concatenate)(w436, w435) -> (w439:string[])
            }
            n225 = local write "Sub-Cycle Pattern"(w428) -> ()
          }
        }
      }
      frame "delete subc" {
        n226 = Two Button Dialog(message="This operation will permanently delete this file!\nDo you want to continue?") -> (T button?=w450:bool)  [unwired: 2 in]
        n227 = case shown="True" w450 {
          tunnel: w451 -> [_ w456]
          frame False {
          }
          frame True {
            n228 = local read "Sub-Cycle List"() -> (w453:i32)
            n229 = property on="Sub-Cycle List" class="LstBox (strict)"() -> ("Item Names"=w454:string[])  [unwired: 2 in, 2 out]
            n230 = Index Array(array=w454, index=w453) -> (element=w458:string)
            n231 = Concatenate Strings(w456, w458) -> (w457:string)
            n232 = local write "Flag1"(FALSE) -> ()
            n233 = String To Path(string=w457) -> (path=w455:path)
            n234 = Delete(path (use dialog)=w455) -> ()  [unwired: 4 in, 3 out]
          }
        }
      }
      frame "clear table 2" {
        n235 = property on="Cycle Name" class="Str"("Value"="" ("Subcycle name")) -> ()  [unwired: 2 in, 2 out]
        n236 = local write "Flag 2"(FALSE) -> ()
        n237 = local write "Cycle Pattern"(string[][] [["", "", "", "", ""], ["", "", "", "", ""], ["", "", "", "", ""], ["", "", "", "", ""], ["", "", "", "", ""], ["", "", "", "", ""], ["", "", "", "", ""], ["", "", "", "", ""], ["", "", "", "", ""], ["", "", "", "", ""], ["", "", "", "", ""], ["", "", "", "", ""], ["", "", "", "", ""], ["", "", "", "", ""], ["", "", "", "", ""], ["", "", "", "", ""], ["", "", "", "", ""], ["", "", "", "", ""], ["", "", "", "", ""], ["", "", "", "", ""], ["", "", "", "", ""], ["", "", "", "", ""], ["", "", "", "", ""], ["", "", "", "", ""], ["", "", "", "", ""], ["", "", "", "", ""], ["", "", "", "", ""], ["", "", "", "", ""], ["", "", "", "", ""], ["", "", "", "", ""], ["", "", "", "", ""]]) -> ()
      }
      frame "update list 2" {
        n238 = String To Path(string=w464) -> (path=w465:path)
        n239 = List Folder(path=w465, pattern="*.eyec") -> (filenames=w463:string[])  [unwired: 2 in, 3 out]
        n240 = property on="Cycle List" class="LstBox (strict)"("Item Names"=w463) -> ()  [unwired: 2 in, 2 out]
      }
      frame "save cycle" {
        w466 = ".eyec" ("string")
        n241 = local read "Cycle Name"() -> (w467:T5)
        n242 = String To Path(string=w479) -> (path=w480:path)
        n243 = List Folder(path=w480, pattern="*.eyec" ("string")) -> (filenames=w478:string[])  [unwired: 2 in, 3 out]
        n244 = Equal?(x=w467, y="") -> (x = y?=w473:bool)
        n245 = Concatenate Strings(w467, w466) -> (w469:string)
        n246 = Search 1D Array(1D array=w478, element=w469) -> (index of element=w477:i32)  [unwired: 1 in]
        n247 = Concatenate Strings(w479, w467, w466) -> (w482:string)
        n248 = case shown="True" w473 {
          tunnel: [TRUE FALSE] -> w471
          frame False {
          }
          frame True {
            n249 = One Button Dialog(message="Insert file name!") -> ()  [unwired: 1 in, 1 out]
          }
        }
        n250 = String To Path(string=w482) -> (path=w481:path)
        n251 = Equal?(x=w477, y=-1) -> (x = y?=w475:bool)
        n252 = case shown="False" w475 {
          selector: w475 -> [_ w531]
          tunnel: [w529 w531] -> w472
          frame False {
            n253 = Two Button Dialog(message="A file with this name already exists!\nDo you want to overwrite?") -> (T button?=w529:bool)  [unwired: 2 in]
          }
          frame True {
          }
        }
        n254 = And(x=w472, y=w471) -> (x .and. y?=w470:bool)
        n255 = case shown="True" w470 {
          tunnel: w481 -> [_ w489]
          frame False {
          }
          frame True {
            n256 = local read "Cycle Pattern"() -> (w488:string[][])
            n257 = call "Table check.vi"("Input table"=w488) -> ("Incomplete?"=w486:bool, "Length"=w487:i32)  [unwired: 9 in]
            n258 = case shown="False" w486 {
              tunnel: w489 -> [w498 _]
              tunnel: w488 -> [w497 _]
              tunnel: w487 -> [w490 _]
              frame False {
                n259 = Number To Decimal String(number=w490) -> (decimal integer string=w493:string)  [unwired: 1 in]
                n260 = for {
                  N: w490 -> [_]
                  tunnel: w497 -> [w527]
                  shift-right: [w515] -> w494
                  shift-left: string[] [] -> [w525]
                  i -> [w526]
                  w506 = 12 ("length")
                  n261 = Index Array(array=w527, index (row)=w526) -> (element=w521:string[])  [unwired: 1 in]
                  n262 = Index Array(array=w521, index=3) -> (element=w511:string)
                  n263 = Index Array(array=w521, index=1) -> (element=w510:string)
                  n264 = Concatenate Strings("C:\\Setup Files\\Subcycles Folder\\", w510) -> (w522:string)
                  n265 = String To Path(string=w522) -> (path=w523:path)
                  n266 = call-poly <vilib>:"Read From Spreadsheet File.vi"("file path (dialog if empty)"=w523) -> ("first row"=w514:string[])  [unwired: 6 in, 4 out]
                  n267 = Delete From Array(array=w514, length=1, index=0) -> (array with subset deleted=w508:string[])  [unwired: 1 out]
                  n268 = String Length(string=w508) -> (length=w517:i32[])
                  n269 = Array Size(array=w517) -> (size(s)=w509:i32)
                  n270 = Divide(x=w509, y=w506) -> (x/y=w507:dbl)
                  n271 = Decrement(x=w507) -> (x-1=w499:dbl)
                  n272 = Multiply(x=w506, y=w499) -> (x*y=w505:dbl)
                  n273 = Number To Decimal String(number=w499) -> (decimal integer string=w516:string)  [unwired: 1 in]
                  n274 = Delete From Array(array=w508, length=12, index=w505) -> (deleted portion=w502:string[], array with subset deleted=w503:string[])
                  n275 = Index Array(array=w502, index=0) -> (element=w500:string)
                  n276 = Build Array (concatenate)(w510, w511, w516, w500, w503) -> (w520:string[])
                  n277 = Build Array (concatenate)(w525, w520) -> (w515:string[])
                }
                n278 = local write "Flag 2"(FALSE) -> ()
                n279 = Build Array (concatenate)("Cycle Data File for EYECAT - do not modify", w493, w494) -> (w495:string[])
                n280 = call-poly <vilib>:"Write To Spreadsheet File.vi"("1D data"=w495, "file path (dialog if empty)"=w498) -> ()  [unwired: 6 in, 1 out]
              }
              frame True {
                n281 = One Button Dialog(message="The table is incomplete!\nplease review and save again!") -> ()  [unwired: 1 in, 1 out]
              }
            }
          }
        }
      }
      frame "load cycle" {
        n282 = local read "Flag 2"() -> (w535:bool)
        n283 = case shown="True" w535 {
          tunnel: [w574 w576] -> w532
          tunnel: w534 -> [w574 w576]
          tunnel: [TRUE ("T button?") w575] -> w533
          frame False {
          }
          frame True {
            n284 = Two Button Dialog(message="The table has been modified.\nDo you want to continue?") -> (T button?=w575:bool)  [unwired: 2 in]
          }
        }
        n285 = case shown="True" w533 {
          tunnel: w532 -> [_ w538]
          frame False {
          }
          frame True {
            n286 = property on="Cycle List" class="LstBox (strict)"() -> ("Item Names"=w554:string[])  [unwired: 2 in, 2 out]
            n287 = Index Array(array=w554, index="Cycle List") -> (element=w540:string)
            n288 = Concatenate Strings(w538, w540) -> (w553:string)
            n289 = Search/Split String(string=w540, search string/char (-)=".") -> (substring before match=w539:string)  [unwired: 1 in, 2 out]
            n290 = String To Path(string=w553) -> (path=w552:path)
            n291 = local write "Cycle Name"(w539) -> ()
            n292 = call-poly <vilib>:"Read From Spreadsheet File.vi"("file path (dialog if empty)"=w552) -> ("first row"=w536:string[])  [unwired: 6 in, 4 out]
            n293 = Delete From Array(array=w536, length=2, index=0) -> (array with subset deleted=w537:string[])  [unwired: 1 out]
            n294 = Index Array(array=w536, index=1) -> (element=w551:string)
            n295 = Decimal String To Number(string=w551) -> (number=w550:i32)  [unwired: 2 in, 1 out]
            n296 = for {
              N: w550 -> [_]
              tunnel: w537 -> [w572]
              tunnel: [w567] -> w545 mode=indexing
              shift-right: [w557] -> _
              shift-left: 0 ("x") -> [w558]
              i -> [w571]
              w568 = ""
              n297 = Increment(x=w558) -> (x+1=w556:i32)
              n298 = Increment(x=w556) -> (x+1=w564:i32)
              n299 = Increment(x=w571) -> (x+1=w566:i32)
              n300 = Number To Decimal String(number=w566) -> (decimal integer string=w565:string)  [unwired: 1 in]
              n301 = Index Array(array=w572, index #1=w558, index #2=w556, index #3=w564) -> (element #1=w570:string, element #2=w569:string, element #3=w563:string)
              n302 = Build Array(w565, w570, w568, w569, w568) -> (w567:string[])
              n303 = Decimal String To Number(string=w563) -> (number=w562:i32)  [unwired: 2 in, 1 out]
              n304 = Multiply(x=w562, y=12 ("x")) -> (x*y=w560:i32)
              n305 = Compound Arithmetic op=ADD(w560, 4, w558) -> (w557:i32)
            }
            n306 = Insert Into Array(array=string[][] [["", "", "", "", ""], ["", "", "", "", ""], ["", "", "", "", ""], ["", "", "", "", ""], ["", "", "", "", ""], ["", "", "", "", ""], ["", "", "", "", ""], ["", "", "", "", ""], ["", "", "", "", ""], ["", "", "", "", ""], ["", "", "", "", ""], ["", "", "", "", ""], ["", "", "", "", ""], ["", "", "", "", ""], ["", "", "", "", ""], ["", "", "", "", ""], ["", "", "", "", ""], ["", "", "", "", ""], ["", "", "", "", ""], ["", "", "", "", ""], ["", "", "", "", ""], ["", "", "", "", ""], ["", "", "", "", ""], ["", "", "", "", ""], ["", "", "", "", ""], ["", "", "", "", ""], ["", "", "", "", ""], ["", "", "", "", ""], ["", "", "", "", ""], ["", "", "", "", ""], ["", "", "", "", ""]], index (row)=0, new element=w545) -> (w544:string[][])  [unwired: 1 in]
            n307 = local write "Cycle Pattern"(w544) -> ()
          }
        }
      }
      frame "delete cycle" {
        n308 = Two Button Dialog(message="This operation will permanently delete this file!\nDo you want to continue?") -> (T button?=w580:bool)  [unwired: 2 in]
        n309 = case shown="True" w580 {
          tunnel: w579 -> [_ w585]
          frame False {
          }
          frame True {
            n310 = local read "Cycle List"() -> (w586:i32)
            n311 = property on="Cycle List" class="LstBox (strict)"() -> ("Item Names"=w587:string[])  [unwired: 2 in, 2 out]
            n312 = Index Array(array=w587, index=w586) -> (element=w584:string)
            n313 = Concatenate Strings(w585, w584) -> (w583:string)
            n314 = String To Path(string=w583) -> (path=w582:path)
            n315 = Delete(path (use dialog)=w582) -> ()  [unwired: 4 in, 3 out]
            n316 = local write "Flag 2"(FALSE) -> ()
          }
        }
      }
      frame "calc HC CO" {
        n317 = local read "Sub-Cycle Pattern"() -> (w604:string[][])
        n318 = Index Array(array=w604, index (col) #1=3 ("disabled index (col)"), index (col) #2=4 ("index (col)"), index (col) #3=11 ("index (col)")) -> (element #1=w594:string[], element #2=w601:string[], element #3=w588:string[])  [unwired: 3 in]
        n319 = Array Size(array=w594) -> (size(s)=w592:i32)
        n320 = Search 1D Array(1D array=w594, element="") -> (index of element=w591:i32)  [unwired: 1 in]
        n321 = Equal?(x=w591, y=-1) -> (x = y?=w593:bool)
        n322 = Select(t=w592, s=w593, f=w591) -> (s? t:f=w590:i32)
        n323 = for {
          N: w590 -> [_]
          tunnel: [w615] -> w598 mode=indexing
          tunnel: [w614] -> w597 mode=indexing
          tunnel: w594 -> [w613] mode=indexing
          tunnel: w601 -> [w612] mode=indexing
          tunnel: w588 -> [w611] mode=indexing
          w610 = ""
          n324 = Not Equal?(x=w613, y=w610) -> (x != y?=w609:bool)
          n325 = Not Equal?(x=w612, y=w610) -> (x != y?=w608:bool)
          n326 = Not Equal?(x=w611, y=w610) -> (x != y?=w607:bool)
          n327 = Compound Arithmetic op=AND(w609, w608, w607) -> (w606:bool)
          n328 = case shown="True" w606 {
            tunnel: w613 -> [_ w644]
            tunnel: w612 -> [_ w643]
            tunnel: [w616 w640] -> w614
            tunnel: [w616 w639] -> w615
            tunnel: w611 -> [_ w617]
            frame False {
              w616 = ""
            }
            frame True {
              # "O2Eq"
              n329 = Fract/Exp String To Number(string=w617) -> (number=w618:dbl)  [unwired: 3 in, 1 out]
              n330 = Fract/Exp String To Number(string=w644) -> (number=w625:dbl)  [unwired: 3 in, 1 out]
              n331 = Fract/Exp String To Number(string=w643) -> (number=w621:dbl)  [unwired: 3 in, 1 out]
              n332 = Decrement(x=w625) -> (x-1=w626:dbl)
              n333 = Divide(x=w618, y=20000.0) -> (x/y=w619:dbl)
              n334 = Multiply(x=4.76, y=w625) -> (x*y=w630:dbl)
              n335 = Multiply(x=w626, y=100.0) -> (x*y=w628:dbl)
              n336 = Add(x=w621, y=w619) -> (x+y=w622:dbl)
              n337 = Add(x=0.33, y=w630) -> (x+y=w632:dbl)
              n338 = Divide(x=w628, y=w632) -> (x/y=w633:dbl)
              n339 = Subtract(x=w622, y=w633) -> (x-y=w635:dbl)
              n340 = Multiply(x=w635, y=2.0) -> (x*y=w623:dbl)
              n341 = Divide(x=w635, y=5.0) -> (x/y=w624:dbl)
              n342 = Number To Fractional String(number=w624, width (-)=i16 6, precision (6)=i16 3) -> (F-format string=w639:string)  [unwired: 1 in]
              n343 = Number To Fractional String(number=w623, width (-)=i16 6, precision (6)=i16 2) -> (F-format string=w640:string)  [unwired: 1 in]
            }
          }
        }
        n344 = Replace Array Subset(array=w604, new element #1=w598, index (col) #1=5 ("disabled index (col)"), new element #2=w597, index (col) #2=6 ("disabled index (col)")) -> (w602:string[][])  [unwired: 2 in]
        n345 = local write "Sub-Cycle Pattern"(w602) -> ()
      }
      frame "Total time calc" {
        w659 = i16 2 ("width (-)")
        w666 = ":"
        n346 = local read "Cycle Pattern"() -> (w673:string[][])
        n347 = Index Array(array=w673, index (col)=4 ("disabled index (col)")) -> (element=w646:string[])  [unwired: 1 in]
        n348 = Array Size(array=w646) -> (size(s)=w648:i32)
        n349 = Search 1D Array(1D array=w646, element="") -> (index of element=w647:i32)  [unwired: 1 in]
        n350 = Equal?(x=w647, y=-1) -> (x = y?=w649:bool)
        n351 = Select(t=w648, s=w649, f=w647) -> (s? t:f=w645:i32)
        n352 = for {
          N: w645 -> [_]
          tunnel: w646 -> [w681] mode=indexing
          shift-right: [w683] -> w669
          shift-left: 0 -> [w684]
          n353 = xnode "Match Regular Expression"("input string"=w681, "regular expression"=":" ("search string/char (-)")) -> ("before match"=w680:string, "after match"=w677:string)  [unwired: 4 in, 3 out]
          n354 = Decimal String To Number(string=w680) -> (number=w679:i32)  [unwired: 2 in, 1 out]
          n355 = Decimal String To Number(string=w677) -> (number=w676:i32)  [unwired: 2 in, 1 out]
          n356 = Multiply(x=w679, y=60) -> (x*y=w675:i32)
          n357 = Add(x=w675, y=w676) -> (x+y=w674:i32)
          n358 = Add(x=w674, y=w684) -> (x+y=w683:i32)
        }
        n359 = local read "Total Number of Cycles"() -> (w670:T1)
        n360 = Multiply(x=w669, y=w670) -> (x*y=w665:T1)
        n361 = Quotient & Remainder(x=w665, y=3600.0) -> (x-y*floor(x/y)=w652:T1, floor(x/y)=w662:T1)
        n362 = Quotient & Remainder(x=w652, y=60.0) -> (x-y*floor(x/y)=w660:T1, floor(x/y)=w661:T1)
        n363 = Number To Decimal String(number=w662) -> (decimal integer string=w667:string)  [unwired: 1 in]
        n364 = Number To Decimal String(number=w661, width (-)=w659) -> (decimal integer string=w663:string)
        n365 = Number To Decimal String(number=w660, width (-)=w659) -> (decimal integer string=w658:string)
        n366 = Concatenate Strings(w667, w666, w663, w666, w658) -> (w657:string)
        n367 = call <vilib>:"Search and Replace Pattern.vi"("string"=w657, "regular expression (\"\")"=" " ("replace string (\"\")"), "replace string (\"\")"="0" ("replace string (\"\")"), "replace all? (F)"=TRUE) -> ("result string"=→"Total Test Duration (hrs)":string)  [unwired: 1 in, 1 out]
      }
      frame "update Cycle pattern " {
        n368 = local read "Cycle Pattern"() -> (w812:string[][])
        n369 = Index Array(array=w812, index (col)=1 ("disabled index (col)")) -> (element=w797:string[])  [unwired: 1 in]
        n370 = String To Path(string=w814) -> (path=w815:path)
        n371 = Array Size(array=w797) -> (size(s)=w800:i32)
        n372 = Search 1D Array(1D array=w797, element="") -> (index of element=w799:i32)  [unwired: 1 in]
        n373 = List Folder(path=w815, pattern="*.eyes") -> (filenames=w813:string[])  [unwired: 2 in, 3 out]
        n374 = Equal?(x=w799, y=-1) -> (x = y?=w801:bool)
        n375 = Select(t=w800, s=w801, f=w799) -> (s? t:f=w798:i32)
        n376 = for {
          N: w798 -> [_]
          tunnel: w812 -> [w831] mode=indexing
          tunnel: w814 -> [w824]
          tunnel: [w826] -> w807 mode=indexing
          tunnel: [w828] -> w811 mode=indexing
          tunnel: [w825] -> w808 mode=indexing
          tunnel: w813 -> [w823]
          tunnel: [w818] -> w804 mode=indexing
          n377 = Index Array(array=w831, index #1=1 ("index"), index #2=3 ("index")) -> (element #1=w822:string, element #2=w827:string)
          n378 = Search 1D Array(1D array=w823, element=w822) -> (index of element=w821:i32)  [unwired: 1 in]
          n379 = Not Equal?(x=w821, y=-1) -> (x != y?=w819:bool)
          n380 = case shown="True" w819 {
            tunnel: [w835 w849] -> w828
            tunnel: w827 -> [_ w845]
            tunnel: [w835 w843] -> w826
            tunnel: [w835 w842] -> w825
            tunnel: w824 -> [_ w841]
            tunnel: w822 -> [w834 w840]
            tunnel: [w833 w840] -> w818
            frame False {
              w835 = "N/A" ("String")
              n381 = Concatenate Strings(w834, " - File NOT AVAILABLE !!!" ("string")) -> (w833:string)
            }
            frame True {
              w853 = i16 2 ("width (-)")
              n382 = Concatenate Strings(w841, w840) -> (w871:string)
              n383 = String To Path(string=w871) -> (path=w870:path)
              n384 = call <vilib>:"Search and Replace Pattern.vi"("string"=w845, "regular expression (\"\")"="[a-x ]" ("format string"), "replace string (\"\")"="", "replace all? (F)"=TRUE) -> ("result string"=w842:string)  [unwired: 1 in, 1 out]
              n385 = call-poly <vilib>:"Read From Spreadsheet File.vi"("file path (dialog if empty)"=w870) -> ("first row"=w839:string[])  [unwired: 6 in, 4 out]
              n386 = Delete From Array(array=w839, length=1, index=0) -> (array with subset deleted=w838:string[])  [unwired: 1 out]
              n387 = Array Size(array=w838) -> (size(s)=w869:i32)
              n388 = Equal?(x=w842, y="") -> (x = y?=w857:bool)
              n389 = Subtract(x=w869, y=12) -> (x-y=w867:i32)
              n390 = Select(t="0", s=w857, f=w842) -> (s? t:f=w856:string)
              n391 = Index Array(array=w838, index=w867) -> (element=w843:string)
              n392 = Decimal String To Number(string=w856) -> (number=w866:i32)  [unwired: 2 in, 1 out]
              n393 = Decimal String To Number(string=w843) -> (number=w865:i32)  [unwired: 2 in, 1 out]
              n394 = Multiply(x=w866, y=w865) -> (x*y=w864:i32)
              n395 = Quotient & Remainder(x=w864, y=60) -> (x-y*floor(x/y)=w862:i32, floor(x/y)=w861:i32)
              n396 = Number To Decimal String(number=w862, width (-)=w853) -> (decimal integer string=w859:string)
              n397 = Number To Decimal String(number=w861, width (-)=w853) -> (decimal integer string=w858:string)
              n398 = Concatenate Strings(w858, ":", w859) -> (w852:string)
              n399 = call <vilib>:"Search and Replace Pattern.vi"("string"=w852, "regular expression (\"\")"=" " ("replace string (\"\")"), "replace string (\"\")"="0" ("replace string (\"\")"), "replace all? (F)"=TRUE) -> ("result string"=w849:string)  [unwired: 1 in, 1 out]
            }
          }
        }
        n400 = Replace Array Subset(array=w812, new element #1=w804, index (col) #1=1 ("disabled index (col)"), new element #2=w807, index (col) #2=2 ("disabled index (col)"), new element #3=w808, index (col) #3=3 ("disabled index (col)"), new element #4=w811, index (col) #4=4 ("disabled index (col)")) -> (w816:string[][])  [unwired: 4 in]
        n401 = local write "Cycle Pattern"(w816) -> ()
      }
      frame "load cycle name" {
        n402 = property on="Cycle Pattern" class="Tbl (strict)"() -> ("EditPos"=w877:T3)  [unwired: 2 in, 2 out]
        n403 = Unbundle By Name(w877) -> ("Row"=w875:i32, "Column"=w874:i32)
        n404 = local read "Cycle Pattern"() -> (w873:string[][])
        n405 = call "SubCycles list.vi"() -> ("Subcycle name"=w876:string)  [unwired: 10 in, 1 out]
        n406 = Replace Array Subset(array=w873, new element=w876, index (row)=w875, index (col)=w874) -> (w872:string[][])
        n407 = local write "Cycle Pattern"(w872) -> ()
      }
      frame "load test array" {
        n408 = local read "Total Test Duration (hrs)"() -> (w885:T8)
        n409 = local read "Cycle Name"() -> (w881:T5)
        n410 = Equal?(x=w881, y="") -> (x = y?=w880:bool)
        n411 = Not Equal?(x=w885, y="0:00:00") -> (x != y?=w879:bool)
        n412 = Or(x=w879, y=w880) -> (x .or. y?=w878:bool)
        n413 = case shown="True" w878 {
          selector: w878 -> [w886 _]
          tunnel: [FALSE TRUE] -> w883
          frame False {
            n414 = case shown="False" w886 {
              frame False {
                n415 = One Button Dialog(message="Incomplete Data!\nReview the cycle pattern!") -> ()  [unwired: 1 in, 1 out]
              }
              frame True {
              }
            }
          }
          frame True {
            w892 = 0.0 ("default (0 I32)")
            n416 = local read "Cycle Name"() -> (w907:T5)
            n417 = Concatenate Strings("C:\\Setup Files\\Cycles Folder\\", w907, ".eyec" ("string")) -> (w905:string)
            n418 = String To Path(string=w905) -> (path=w906:path)
            n419 = local read "Total Number of Cycles"() -> (w903:T1)
            n420 = call-poly <vilib>:"Read From Spreadsheet File.vi"("file path (dialog if empty)"=w906) -> ("first row"=w889:string[])  [unwired: 6 in, 4 out]
            n421 = call "Remove names.vi"("Array in"=w889) -> ("Array out"=w898:string[])  [unwired: 10 in]
            n422 = Index Array(array=w889, index #1=14 ("index"), index #2=15 ("index")) -> (element #1=w894:string, element #2=w890:string)
            n423 = Number To Decimal String(number="Ageing Gas") -> (decimal integer string=w902:string)  [unwired: 1 in]
            n424 = Number To Decimal String(number=w903) -> (decimal integer string=w901:string)  [unwired: 1 in]
            n425 = Decimal String To Number(string=w890, default (0L)=w892) -> (number=w891:dbl)  [unwired: 1 in, 1 out]
            n426 = Decimal String To Number(string=w894, default (0L)=w892) -> (number=w893:dbl)  [unwired: 1 in, 1 out]
            n427 = property on="Inlet temp Age" class="DigNum (strict)"("Value"=w893) -> ()  [unwired: 2 in, 2 out]
            n428 = property on="Flow rate Age" class="DigNum (strict)"("Value"=w891) -> ()  [unwired: 2 in, 2 out]
            n429 = Build Array (concatenate)(w902, w901, w898) -> (w897:string[])
            n430 = shared-variable "NI-cRIO9074-018C1D8D\\Library 1.lvlib\\Ageing Variables"(w897) -> ()  [unwired: 1 in, 1 out]
          }
        }
        "Test Compiled" <- w883
      }
      frame "convert to num" {
        n431 = local read "EditPos Subc"() -> (w912:T3)
        n432 = Unbundle By Name(w912) -> ("Row"=w913:i32, "Column"=w910:i32)
        n433 = Equal?(x=w910, y=7) -> (x = y?=w909:bool)
        n434 = case shown="False" w909 {
          tunnel: w913 -> [_ w918]
          tunnel: w910 -> [_ w916]
          tunnel: w912 -> [_ _]
          frame True {
          }
          frame False {
            n435 = local read "Sub-Cycle Pattern"() -> (w915:string[][])
            n436 = call "Conv to num.vi"("Column"=w916, "Row"=w918, "Array"=w915) -> ("result string"=w917:string)  [unwired: 8 in]
            n437 = Replace Array Subset(array=w915, new element=w917, index (row)=w918, index (col)=w916) -> (w914:string[][])
            n438 = local write "Sub-Cycle Pattern"(w914) -> ()
          }
        }
      }
      frame "check scycle name" {
        n439 = local read "Sub-Cycle Name"() -> (w919:T5)
        n440 = call <vilib>:"Search and Replace Pattern.vi"("string"=w919, "regular expression (\"\")"="[^0-9a-zA-Z ]" ("format string"), "replace string (\"\")"="", "replace all? (F)"=TRUE) -> ("result string"=w925:string)  [unwired: 1 in, 1 out]
        n441 = Not Equal?(x=w925, y=w919) -> (x != y?=w924:bool)
        n442 = case shown="False" w924 {
          tunnel: w925 -> [w926 w927]
          tunnel: [w926 w927] -> w920
          frame False {
          }
          frame True {
            n443 = One Button Dialog(message="Unsuitable character for the file name!") -> ()  [unwired: 1 in, 1 out]
          }
        }
        n444 = local write "Sub-Cycle Name"(w920) -> ()
      }
      frame "check cycle name" {
        n445 = local read "Cycle Name"() -> (w929:T5)
        n446 = call <vilib>:"Search and Replace Pattern.vi"("string"=w929, "regular expression (\"\")"="[^0-9a-zA-Z ]" ("format string"), "replace string (\"\")"="", "replace all? (F)"=TRUE) -> ("result string"=w935:string)  [unwired: 1 in, 1 out]
        n447 = Not Equal?(x=w935, y=w929) -> (x != y?=w934:bool)
        n448 = case shown="False" w934 {
          tunnel: w935 -> [w936 w937]
          tunnel: [w936 w937] -> w930
          frame False {
          }
          frame True {
            n449 = One Button Dialog(message="Unsuitable character for the file name!") -> ()  [unwired: 1 in, 1 out]
          }
        }
        n450 = local write "Cycle Name"(w930) -> ()
      }
      frame "Multigas connect" {
        n451 = flat-sequence {
          frame #0 {
            "Connected?" <- TRUE
          }
        }
      }
      frame "Multigas disconnect" {
      }
    }
    n452 = local read "stop 2"() -> (w325:bool)
  }
  n453 = disable-structure shown="Disabled" {
    frame Disabled {
      n454 = while {
        tunnel: [w978] -> w963
        tunnel: [w977] -> w962
        stop <- w974 stop-if-true
        n455 = TCP Open Connection(address="192.168.1.3", remote port or service name=u16 7700) -> (connection ID=w978:refnum<k5>, error out=w977:errorcluster)  [unwired: 3 in]
        n456 = Unbundle By Name(w977) -> ("status"=w979:bool)
        n457 = Not(x=w979) -> (.not. x?=w975:bool)
        n458 = Or(x=w975, y="stop TCP") -> (x .or. y?=w974:bool)
      }
      n459 = Concatenate Strings("\r", "\n") -> (w951:string)
      n460 = Concatenate Strings("MSSM,0,1,1" ("data in"), w951) -> (w958:string)
      n461 = TCP Write(connection ID=w963, data in=w958, error in (no error)=w962) -> (connection ID out=w966:refnum<k5>, error out=w967:errorcluster)  [unwired: 1 in, 1 out]
      n462 = Concatenate Strings("MSMD,1,7,1,1,1,1,2,1,1,3,1,1,4,1,1,5,1,1,6,1,1,7,1" ("data in"), w951) -> (w953:string)
      n463 = TCP Write(connection ID=w966, data in=w953, error in (no error)=w967) -> (connection ID out=w964:refnum<k5>, error out=w965:errorcluster)  [unwired: 1 in, 1 out]
      n464 = Concatenate Strings("MSTT,1,0" ("string"), w951) -> (w952:string)
      n465 = TCP Write(connection ID=w964, data in=w952, error in (no error)=w965) -> (connection ID out=w950:refnum<k5>, error out=w949:errorcluster)  [unwired: 1 in, 1 out]
      n466 = UDP Open(9:500 ("timeout ms (25000)"), 11:u16 7701 ("port")) -> ()  [unwired: 3 in, 3 out]
      n467 = UDP Read(timeout ms (25000)=500) -> (data out=w941:string)  [unwired: 3 in, 4 out]
      n468 = while {
        shift-right: [w970] -> _
        shift-left: w941 -> [w973]
        tunnel: [w971] -> w942 mode=indexing
        stop <- w968 stop-if-true
        n469 = Search/Split String(string=w973, search string/char (-)=",") -> (substring before match=w971:string, match + rest of string=w970:string)  [unwired: 1 in, 1 out]
        n470 = String Length(string=w970) -> (length=w969:i32)
        n471 = Equal To 0?(x=w969) -> (x = 0?=w968:bool)
      }
      n472 = call "7170string to array.vi"("Array in"=w942) -> ()  [unwired: 4 in, 1 out]
      n473 = UDP Close() -> ()  [unwired: 2 in, 2 out]
      n474 = Concatenate Strings("MSTP,0,0" ("string"), "\r", "\n") -> (w945:string)
      n475 = TCP Write(data in=w945) -> (connection ID out=w947:refnum<k5>, error out=w948:errorcluster)  [unwired: 3 in, 1 out]
      n476 = TCP Close Connection(connection ID=w947, error in (no error)=w948) -> ()  [unwired: 1 in, 2 out]
    }
    frame Enabled {
    }
  }
  n477 = while {
    tunnel: w35 -> [w986]
    shift-right: [w984] -> _
    shift-left: _ -> [w983]
    stop <- w982 stop-if-true
    n478 = event shown="[12] \"Cycle Pattern\": Mouse Up;  \"Cycle Pattern\": Value Change" {
      selector: _ -> [_ _ _ _ _ _ _ _ _ _ _ _ _ _ _ _ _ _ _ _ _ _ _ _ _ _ _ _]
      dyn-events: _ -> [_ _ _ _ _ _ _ _ _ _ _ _ _ _ _ _ _ _ _ _ _ _ _ _ _ _ _ _]
      timeout: 100 -> [_ _ _ _ _ _ _ _ _ _ _ _ _ _ _ _ _ _ _ _ _ _ _ _ _ _ _ _]
      tunnel: w986 -> [w989 w991 _ w1000 w1008 w1015 w1022 w1033 w1037 w1048 w1053 w1056 w1061 w1083 w1091 w1092 _ _ _ _ w1136 w1146 w1168 w1186 _ w1200 _ _]
      tunnel: [w987 w990 _ w1001 w1007 w1014 w1021 w1032 w1035 w1043 w1050 w1055 w1059 w1080 _ _ _ _ _ _ _ _ _ _ _ _ _ _] -> w984
      tunnel: w983 -> [w987 w990 _ w1001 w1007 w1014 w1020 w1032 w1035 w1043 w1050 w1055 w1059 w1080 _ _ _ _ _ _ _ _ _ _ _ _ _ _]
      tunnel: [_ _ w993 _ _ _ _ _ _ _ _ _ _ _ _ _ _ _ _ _ _ _ _ _ _ _ _ _] -> w982
      event Timeout {
        n479 = event-data() -> ()  [unwired: 1 in, 2 out]
        n480 = Enqueue Element(queue=w989, element=Control_3."main" ("Enum")) -> ()  [unwired: 2 in, 3 out]
      }
      event "Clear subcycle": Value Change {
        n481 = event-data() -> ()  [unwired: 1 in, 5 out]
        n482 = Enqueue Element(queue=w991, element=Control_3."clear table 1" ("Enum")) -> ()  [unwired: 2 in, 3 out]
      }
      event Panel Close? {
        n483 = event-data() -> ()  [unwired: 1 in, 3 out]
        n484 = Two Button Dialog(message="This command will close Eyecat!\nDo you wish to continue?", 1:"No" ("F button name (\"Cancel\")"), 2:"Yes" ("T button name (\"OK\")")) -> (T button?=w993:bool)
        n485 = Not(x=w993) -> (.not. x?=w994:bool)
        n486 = event-data("Discard?"=w994) -> ()  [unwired: 1 in, 1 out]
      }
      event "Save sCycle": Value Change {
        n487 = event-data() -> ()  [unwired: 1 in, 5 out]
        n488 = local read "Sub-Cycle Pattern"() -> (w998:string[][])
        n489 = call "Time column check.vi"("Array"=w998) -> ("Mistake?"=w999:bool)  [unwired: 10 in]
        n490 = case shown="False" w999 {
          tunnel: w1000 -> [w1002 _]
          frame False {
            n491 = Enqueue Element(queue=w1002, element=Control_3."save subc") -> (queue out=w1004:refnum<queue>)  [unwired: 2 in, 2 out]
            n492 = Enqueue Element(queue=w1004, element=Control_3."update list 1") -> ()  [unwired: 2 in, 3 out]
          }
          frame True {
            n493 = One Button Dialog(message="The time sequence is incorrect!\nReview and save again!") -> ()  [unwired: 1 in, 1 out]
          }
        }
      }
      event "Load sCycle": Value Change {
        n494 = event-data() -> ()  [unwired: 1 in, 5 out]
        n495 = Enqueue Element(queue=w1008, element=Control_3."load subc") -> ()  [unwired: 2 in, 3 out]
      }
      event "Delete sCycle": Value Change {
        n496 = event-data() -> ()  [unwired: 1 in, 5 out]
        n497 = Enqueue Element(queue=w1015, element=Control_3."delete subc") -> (queue out=w1017:refnum<queue>)  [unwired: 2 in, 2 out]
        n498 = Enqueue Element(queue=w1017, element=Control_3."update list 1") -> (queue out=w1013:refnum<queue>)  [unwired: 2 in, 2 out]
        n499 = Enqueue Element(queue=w1013, element=Control_3."update Cycle pattern ") -> (queue out=w1010:refnum<queue>)  [unwired: 2 in, 2 out]
        n500 = Enqueue Element(queue=w1010, element=Control_3."Total time calc") -> ()  [unwired: 2 in, 3 out]
      }
      event "Sub-Cycle Pattern": Mouse Down; "Sub-Cycle Pattern": Value Change {
        n501 = event-data() -> ()  [unwired: 1 in, 3 out]
        n502 = property on="Sub-Cycle Pattern" class="Tbl (strict)"() -> ("EditPos"=w1021:T3)  [unwired: 2 in, 2 out]
        n503 = Unbundle By Name(w1021) -> ("Row"=w1023:i32)  [unwired: 1 out]
        n504 = Less?(x=w1023, y=30) -> (x < y?=w1025:bool)
        n505 = case shown="True" w1025 {
          tunnel: w1022 -> [_ w1030]
          frame False {
            n506 = One Button Dialog(message="This table is limited to 30 entries!") -> ()  [unwired: 1 in, 1 out]
          }
          frame True {
            n507 = Enqueue Element(queue=w1030, element=Control_3."convert to num") -> (queue out=w1029:refnum<queue>)  [unwired: 2 in, 2 out]
            n508 = Enqueue Element(queue=w1029, element=Control_3."calc HC CO") -> ()  [unwired: 2 in, 3 out]
          }
        }
        "EditPos Subc" <- w1020
        "Flag1" <- TRUE
      }
      event "Clear Cycle Pattern": Value Change {
        n509 = event-data() -> ()  [unwired: 1 in, 5 out]
        n510 = Enqueue Element(queue=w1033, element=Control_3."clear table 2" ("Enum")) -> ()  [unwired: 2 in, 3 out]
        n511 = local write "Test Compiled"(FALSE ("Test Compiled")) -> ()
      }
      event "Save Cycle": Value Change {
        n512 = event-data() -> ()  [unwired: 1 in, 5 out]
        n513 = Enqueue Element(queue=w1037, element=Control_3."update Cycle pattern ") -> (queue out=w1036:refnum<queue>)  [unwired: 2 in, 2 out]
        n514 = Enqueue Element(queue=w1036, element=Control_3."save cycle") -> (queue out=w1040:refnum<queue>)  [unwired: 2 in, 2 out]
        n515 = Enqueue Element(queue=w1040, element=Control_3."update list 2") -> ()  [unwired: 2 in, 3 out]
      }
      event "Load Cycle": Value Change {
        n516 = event-data() -> ()  [unwired: 1 in, 5 out]
        n517 = Enqueue Element(queue=w1048, element=Control_3."load cycle") -> (queue out=w1046:refnum<queue>)  [unwired: 2 in, 2 out]
        n518 = Enqueue Element(queue=w1046, element=Control_3."update Cycle pattern ") -> (queue out=w1045:refnum<queue>)  [unwired: 2 in, 2 out]
        n519 = local write "Test Compiled"(FALSE ("Test Compiled")) -> ()
        n520 = Enqueue Element(queue=w1045, element=Control_3."Total time calc") -> ()  [unwired: 2 in, 3 out]
      }
      event "Delete Cycle": Value Change {
        n521 = event-data() -> ()  [unwired: 1 in, 5 out]
        n522 = Enqueue Element(queue=w1053, element=Control_3."delete cycle") -> (queue out=w1052:refnum<queue>)  [unwired: 2 in, 2 out]
        n523 = Enqueue Element(queue=w1052, element=Control_3."update list 2") -> ()  [unwired: 2 in, 3 out]
      }
      event Value Change {
        n524 = event-data() -> ()  [unwired: 1 in, 5 out]
        n525 = Enqueue Element(queue=w1056, element=Control_3."Total time calc") -> ()  [unwired: 2 in, 3 out]
      }
      event "Cycle Pattern": Mouse Up; "Cycle Pattern": Value Change {
        n526 = event-data() -> ()  [unwired: 1 in, 3 out]
        n527 = property on="Cycle Pattern" class="Tbl (strict)"() -> ("EditPos"=w1063:T3)  [unwired: 2 in, 2 out]
        n528 = Unbundle By Name(w1063) -> ("Row"=w1060:i32, "Column"=w1065:i32)
        n529 = Less?(x=w1060, y=30) -> (x < y?=w1064:bool)
        n530 = case shown="True" w1064 {
          tunnel: w1065 -> [_ w1067]
          tunnel: w1061 -> [_ w1070]
          frame False {
            n531 = One Button Dialog(message="This table is limited to 30 entries!") -> ()  [unwired: 1 in, 1 out]
          }
          frame True {
            n532 = Equal?(x=w1067, y=1) -> (x = y?=w1071:bool)
            n533 = case shown="True" w1071 {
              tunnel: w1070 -> [w1074 w1077]
              tunnel: [w1073 w1076] -> w1069
              frame False {
                n534 = Enqueue Element(queue=w1074, element=Control_3."update Cycle pattern ") -> (queue out=w1073:refnum<queue>)  [unwired: 2 in, 2 out]
              }
              frame True {
                n535 = Enqueue Element(queue=w1077, element=Control_3."load cycle name") -> (queue out=w1076:refnum<queue>)  [unwired: 2 in, 2 out]
              }
            }
            n536 = Enqueue Element(queue=w1069, element=Control_3."Total time calc") -> ()  [unwired: 2 in, 3 out]
          }
        }
        "Flag 2" <- TRUE
      }
      event "Compile Test Button": Value Change {
        n537 = event-data() -> ()  [unwired: 1 in, 5 out]
        n538 = local read "Flag 2"() -> (w1079:bool)
        n539 = case shown="True" w1079 {
          tunnel: w1083 -> [w1084 w1088]
          tunnel: [w1084 w1085] -> w1081
          frame False {
          }
          frame True {
            n540 = Enqueue Element(queue=w1088, element=Control_3."save cycle") -> (queue out=w1086:refnum<queue>)  [unwired: 2 in, 2 out]
            n541 = Enqueue Element(queue=w1086, element=Control_3."update list 2") -> (queue out=w1085:refnum<queue>)  [unwired: 2 in, 2 out]
          }
        }
        n542 = Enqueue Element(queue=w1081, element=Control_3."load test array") -> ()  [unwired: 2 in, 3 out]
      }
      event Value Change {
        n543 = event-data() -> ()  [unwired: 1 in, 5 out]
        n544 = Enqueue Element(queue=w1091, element=Control_3."check scycle name") -> ()  [unwired: 2 in, 3 out]
      }
      event Value Change {
        n545 = event-data() -> ()  [unwired: 1 in, 5 out]
        n546 = Enqueue Element(queue=w1092, element=Control_3."check cycle name") -> ()  [unwired: 2 in, 3 out]
      }
      event Value Change {
        n547 = event-data() -> ()  [unwired: 1 in, 5 out]
        n548 = Square(x="Sample Diameter (mm)") -> (x^2=w1101:T1)
        n549 = Compound Arithmetic op=MULTIPLY(w1101, "Sample Length (mm)", "Number of Samples", 3.141592653589793) -> (w1100:T1)
        n550 = Divide(x=w1100, y=4000000.0) -> (x/y=→"Sample Volume (litres)":T1)
      }
      event Value Change {
        # "O2Eq"
        n551 = event-data() -> ()  [unwired: 1 in, 5 out]
        n552 = local write "Inlet LAMBDA"("Inlet LAMBDA") -> ()
        n553 = local write "Inlet O2 (%)"("Inlet O2 (%)") -> ()
        n554 = Decrement(x="Inlet LAMBDA") -> (x-1=w1116:T1)
        n555 = Multiply(x=4.76, y="Inlet LAMBDA") -> (x*y=w1112:T1)
        n556 = Multiply(x=w1116, y=100.0) -> (x*y=w1114:T1)
        n557 = Add(x=0.33, y=w1112) -> (x+y=w1110:T1)
        n558 = Divide(x=w1114, y=w1110) -> (x/y=w1109:T1)
        n559 = Subtract(x="Inlet O2 (%)", y=w1109) -> (x-y=w1107:T1)
        n560 = Multiply(x=w1107, y=2.0) -> (x*y=→"CO Theory (%)":T1)
        n561 = Divide(x=w1107, y=4.5) -> (x/y=→"HC Theory (%)":T1)
      }
      event Value Change {
        n562 = event-data() -> ()  [unwired: 1 in, 5 out]
        n563 = local write "NO ppm Loff"("NO ppm Loff") -> ()
        n564 = local write "NO:CO Ratio"("NO:CO Ratio") -> ()
        n565 = Divide(x="NO ppm Loff", y=T1 10000.0) -> (x/y=w1119:T1)
        n566 = Multiply(x="NO:CO Ratio", y=w1119) -> (x*y=→"CO Theory (%)":T1)
      }
      event Value Change {
        n567 = event-data() -> ()  [unwired: 1 in, 5 out]
        n568 = local read "Sample Volume (litres)"() -> (w1124:T7)
        n569 = Equal?(x=w1124, y=0.0) -> (x = y?=w1123:bool)
        n570 = case shown="False" w1123 {
          tunnel: w1124 -> [w1129 _]
          tunnel: "Test Flow Rate(g/s)" -> [w1126 _]
          frame False {
            w1131 = 60.0 ("y")
            n571 = Multiply(x=w1126, y=w1131) -> (x*y=w1133:T1)
            n572 = Divide(x=w1133, y=1.2) -> (x/y=w1128:T1)
            "Vol Flow @ STP (l/min)" <- w1128
            n573 = Multiply(x=w1128, y=w1131) -> (x*y=w1130:T1)
            n574 = Divide(x=w1130, y=w1129) -> (x/y=→"Space Velocity (h-1)":T1)
          }
          frame True {
            n575 = One Button Dialog(message="Review sample specification first!") -> ()  [unwired: 1 in, 1 out]
          }
        }
      }
      event "Execute Leak Test Button": Value Change {
        n576 = event-data() -> ()  [unwired: 1 in, 5 out]
        n577 = flat-sequence {
          tunnel: w1136 -> [w1139]
          tunnel: [w1139] -> w1135
          tunnel: w1135 -> [w1142]
          frame #0 {
            n578 = local write "Test number"(u16 5) -> ()
            n579 = local write "Enum 1"(u16 3 ("Test number")) -> ()
          }
          frame #1 {
            n580 = Enqueue Element(queue=w1142, element=Control_3."main" ("Enum")) -> (queue out=w1140:refnum<queue>)  [unwired: 2 in, 2 out]
            n581 = Enqueue Element(queue=w1140, element=Control_3."start test" ("Enum")) -> ()  [unwired: 2 in, 3 out]
          }
        }
      }
      event "Start Test Button": Value Change {
        n582 = event-data() -> ()  [unwired: 1 in, 5 out]
        n583 = flat-sequence {
          tunnel: w1146 -> [w1149]
          tunnel: [w1149] -> w1145
          tunnel: w1145 -> [w1153]
          tunnel: [w1150] -> w1144
          tunnel: w1144 -> [w1161]
          frame #0 {
            n584 = local write "Enum 1"(u16 1 ("Test number")) -> ()
            "Test number" <- "Select Test Type"
          }
          frame #1 {
            n585 = Two Button Dialog(message="Do you wish to connect to\nthe external analyser?   \n") -> (T button?=w1151:bool)  [unwired: 2 in]
            n586 = case shown="True" w1151 {
              tunnel: w1153 -> [w1154 w1156]
              tunnel: [w1154 w1155] -> w1150
              frame False {
              }
              frame True {
                n587 = Enqueue Element(queue=w1156, element=Control_3."Multigas connect" ("Enum")) -> (queue out=w1155:refnum<queue>)  [unwired: 2 in, 2 out]
              }
            }
          }
          frame #2 {
            n588 = Enqueue Element(queue=w1161, element=Control_3."main" ("Enum")) -> (queue out=w1159:refnum<queue>)  [unwired: 2 in, 2 out]
            n589 = property on="Stop Test Button" class="Bool"("DisabledEnum"=T13."Enabled" ("Disabled")) -> ()  [unwired: 2 in, 2 out]
            n590 = Enqueue Element(queue=w1159, element=Control_3."start test" ("Enum")) -> ()  [unwired: 2 in, 3 out]
          }
        }
      }
      event "Stop Test Button": Value Change {
        n591 = event-data() -> ()  [unwired: 1 in, 5 out]
        n592 = flat-sequence {
          tunnel: w1168 -> [w1170]
          tunnel: [w1170] -> w1167
          tunnel: [w1169] -> w1165
          tunnel: w1167 -> [w1174]
          tunnel: [w1173] -> w1166
          tunnel: w1165 -> [w1173]
          tunnel: [w1172] -> w1164
          tunnel: w1166 -> [w1178]
          tunnel: w1164 -> [w1177]
          tunnel: [T13."Disabled and Grayed Out" ("Disabled")] -> w1163
          frame #0 {
            n593 = local read "Connected?"() -> (w1169:bool)
            n594 = local write "Stop Cmd"(T1 1.0 ("Stop Cmd")) -> ()
          }
          frame #1 {
            n595 = Enqueue Element(queue=w1174, element=Control_3."main" ("Enum")) -> (queue out=w1172:refnum<queue>)  [unwired: 2 in, 2 out]
          }
          frame #2 {
            n596 = case shown="True" w1178 {
              tunnel: w1177 -> [w1179 w1182]
              tunnel: [w1179 w1181] -> _
              frame False {
              }
              frame True {
                n597 = local write "Connected?"(FALSE ("Connected?")) -> ()
                n598 = Enqueue Element(queue=w1182, element=Control_3."Multigas disconnect" ("Enum")) -> (queue out=w1181:refnum<queue>)  [unwired: 2 in, 2 out]
              }
            }
          }
        }
        n599 = property on="Stop Test Button" class="Bool"("DisabledEnum"=w1163) -> ()  [unwired: 2 in, 2 out]
      }
      event "Stopped?": Value Change {
        n600 = event-data() -> ()  [unwired: 1 in, 5 out]
        n601 = flat-sequence {
          tunnel: w1186 -> [w1190]
          tunnel: [w1189] -> w1185
          tunnel: [w1188] -> w1184
          tunnel: w1185 -> [w1192]
          tunnel: w1184 -> [w1191]
          frame #0 {
            n602 = local read "Connected?"() -> (w1188:bool)
            n603 = Enqueue Element(queue=w1190, element=Control_3."main" ("Enum")) -> (queue out=w1189:refnum<queue>)  [unwired: 2 in, 2 out]
          }
          frame #1 {
            n604 = case shown="True" w1191 {
              tunnel: w1192 -> [_ w1193]
              frame False {
              }
              frame True {
                n605 = local write "Connected?"(FALSE ("Connected?")) -> ()
                n606 = Enqueue Element(queue=w1193, element=Control_3."Multigas disconnect" ("Enum")) -> ()  [unwired: 2 in, 3 out]
              }
            }
          }
        }
      }
      event "Alarm ack": Value Change {
        # "system alarm - set to off"
        n607 = event-data() -> ()  [unwired: 1 in, 5 out]
        n608 = local write "Acknowledge"(TRUE ("Acknowledge")) -> ()
        n609 = property on="Soft Alarm" class="Bool (strict)"("Value"=FALSE ("Acknowledge")) -> ()  [unwired: 2 in, 2 out]
        n610 = property on="Alarm ack" class="Bool"("DisabledEnum"=T13."Disabled and Grayed Out" ("Disabled")) -> ()  [unwired: 2 in, 2 out]
      }
      event "Purge System": Value Change {
        n611 = event-data() -> ()  [unwired: 1 in, 5 out]
        n612 = flat-sequence {
          tunnel: w1200 -> [w1202]
          tunnel: [w1202] -> w1199
          tunnel: w1199 -> [w1203]
          frame #0 {
            n613 = local write "Enum 1"(u16 4 ("Test number")) -> ()
          }
          frame #1 {
            n614 = Enqueue Element(queue=w1203, element=Control_3."start test" ("Enum")) -> ()  [unwired: 2 in, 3 out]
          }
        }
      }
      event "Clear log": Value Change {
        n615 = event-data() -> ()  [unwired: 1 in, 5 out]
        n616 = local write "Table"(string[][] [] ("Table")) -> ()
      }
      event "Advanced settings": Value Change {
        # "To be updated"
        # "SO2 conc\nNOx conc\nCO conc\nHC conc\nBleed ratio N2\nBleed ratio CO2"
        n617 = event-data() -> ()  [unwired: 1 in, 5 out]
        n618 = call "Advanced settings MAX.vi"() -> ("output cluster"=→"output cluster":T14)  [unwired: 1 in]
      }
    }
    "stop 2" <- w982
  }
  n619 = local write "stop 2"(w9) -> ()
  n620 = node-c288(w6) -> ()  [unwired: 1 out]
  "Table" <- string[][] [] ("Table")
